vi "demo.vi"() -> ()   [LabVIEW 2017]
uses:
  globe.vi
  Instance           7 12Saved   demo .vi
  Instance           3 12Saved   demo .vi
  Instance           6 12Saved   demo .vi
  Instance           4 12Saved   demo .vi
  Instance           5 12Saved   demo .vi
  Instance           2 12Saved   demo .vi
  Instance           1 12Saved   demo .vi
  bin/ControlCAN.dll
panel:
  in  "清除定时发送":bool
  in  "定时发送":bool
  out "DBC界面":bool
  in  "DBC发送界面":bool
  in  "设备类型":u32(ring)=1 items=["PCI5121"=1, "PCI9810"=2, "USBCAN1"=3, "USBCAN2"=4, "PCI9820"=5, "PCI5110"=7, "PC104CAN"=11, "CANETUDP"=12, "PCI9840B"=14, "PC104C2"=15, "PCI9820I"=16, "CANETTCP"=17, "PCIE9221"=24, "PCI5010U"=19, "USBCAN_E_U"=20, "USBCAN_2E_U"=21, "CANalyst-II+"=10021, "PCI5020U"=22, "PCIE9120I"=27, "PCIE9110I"=28, "PCIE9140I"=29]
  in  "总线利用率":bool
  in  "索引":u32(ring) items=["0", "1", "2", "3", "4", "5", "6", "7", "8"]
  in  "Radio_Baud(E_U)":bool=TRUE
  in  "寄存器":u32 format="0x%08x"
  in  "Radio_Baud":bool=TRUE
  in  "Baud":u32(ring) caption="波特率" items=["5Kbps", "10Kbps", "20Kbps", "40Kbps", "50Kbps", "80Kbps", "100Kbps", "125Kbps", "200Kbps", "250Kbps", "400Kbps", "500Kbps", "666Kbps", "800Kbps", "1000Kbps"]
  out "VCI_CAN_OBJ_TN":T1(array[cluster])
  out "VCI_CAN_OBJ_RN":T1(array[cluster])
  in  "arraylen":u32
  in  "一次发送帧数":u32
  out "type":u8[](array[numeric])
  in  "本机端口":u32
  in  "本机类型":enum32{"Radio Selection 1", "Radio Selection 2"}(radio)
  in  "CANET 端口":u32
  in  "CANET IP":string
  out "VCI_FILTER_RECORD":cluster{"ExtFrame":u32, "Start":u32, "End":u32}
  in  "e-u-baud":cluster{"数值":u32}
  in  "滤波模式":u32(ring) items=["标准帧滤波", "扩展帧滤波", "禁能滤波"]
  in  "滤波起始ID":u32
  in  "滤波结束ID":u32
  in  "Baud(E_U)":u32(ring) caption="波特率" items=["1000Kbps"=393219, "800Kbps"=393220, "500Kbps"=393223, "250Kbps"=1835016, "125Kbps"=1835025, "100Kbps"=1441827, "50Kbps"=1835052, "20Kbps"=1441971, "10Kbps"=1835232, "5Kbps"=1835457]
  in  "SEND_NCAN":bool
  out "VCI_CAN_OBJ_T_N":T1(array[cluster])
  out "接收缓冲区":u32
  in  "GetStatus":bool
  in  "GetErrorInfo":bool
  in  "GetBoardInfo":bool
  in  "Clear Buffer":bool
  in  "Transmit":bool
  out "VCI_BOARD_INFO":T2
  out "VCI_ERR_INFO":T3
  out "VCI_CAN_STATUS":T4
  in  "模式":u8(ring) items=["正常", "只听"]
  in  "滤波方式":u8(ring) items=["双滤波", "单滤波"]
  in  "BTR1":u8=20 format="0x%02x"
  in  "BTR0":u8 format="0x%02x"
  in  "屏蔽码":u32=4294967295 format="0x%08x"
  in  "验收码":u32 format="0x%08x"
  in  "ID":u32 format="0x%08x"
  in  "数据输入":string
  in  "TREvent":T5={"Tx_Or_Rx"=FALSE, "VCI_CAN_OBJ"={"ID"=0, "TimeStamp"=0, "TimeFlag"=0, "SendType"=1, "RemoteFlag"=0, "ExternFlag"=0, "DataLen"=8, 0, 0, 0, 0, 0, 0, 0, 0, 0, 0, 0}, "VCI_CAN_OBJ_N"=[], "Num"=0}
  out "stop 2":bool
  out "Num Rows":u32
  out "TRCount":u32
  out "VCI_CAN_OBJ_R":T6={"ID"=0, "TimeStamp"=0, "TimeFlag"=0, "SendType"=1, "RemoteFlag"=0, "ExternFlag"=0, "DataLen"=8, 0, 0, 0, 0, 0, 0, 0, 0, 0, 0, 0}
  out "VCI_CAN_OBJ_T":T6={"ID"=0, "TimeStamp"=0, "TimeFlag"=0, "SendType"=1, "RemoteFlag"=0, "ExternFlag"=0, "DataLen"=8, 0, 0, 0, 0, 0, 0, 0, 0, 0, 0, 0}
  out "VCI_INIT_CONFIG":T7={"AccCode"=0, "AccMask"=4294967295, "Reserved"=0, "Filter"=1, "Timing0"=0, "Timing1"=20, "Mode"=0}
  out "CANStartup":bool
  in  "DeviceOpen":bool
  in  "OpenDevice":bool
  in  "帧格式":u8(ring) items=["数据帧", "远程帧"]
  in  "帧类型":u8(ring) items=["标准帧", "扩展帧"]
  in  "发送类型":u8(ring) items=["正常发送", "单次发送", "自发自收", "单次自发自收"]
  in  "设备类型值":u32(ring)=1 items=["PCI5121"=1, "PCI9810"=2, "USBCAN1"=3, "USBCAN2"=4, "PCI9820"=5, "PCI5110"=7, "PC104CAN"=11, "CANETUDP"=12, "PCI9840B"=14, "PC104C2"=15, "PCI9820I"=16, "CANETTCP"=17, "PCIE9221"=24, "PCI5010U"=19, "USBCAN_E_U"=20, "USBCAN_2E_U"=21, "PCI5020U"=22, "PCIE9120I"=27, "PCIE9110I"=28, "PCIE9140I"=29]
  in  "ResetCAN":bool
  in  "StartCAN":bool
  in  "CAN 通道":u32(ring) items=["0", "1"]
  in  "stop":bool
  out "Multicolumn Listbox":i32(listbox)
  # "CANET 设备特殊设置"
  # "_U系列特殊设置"
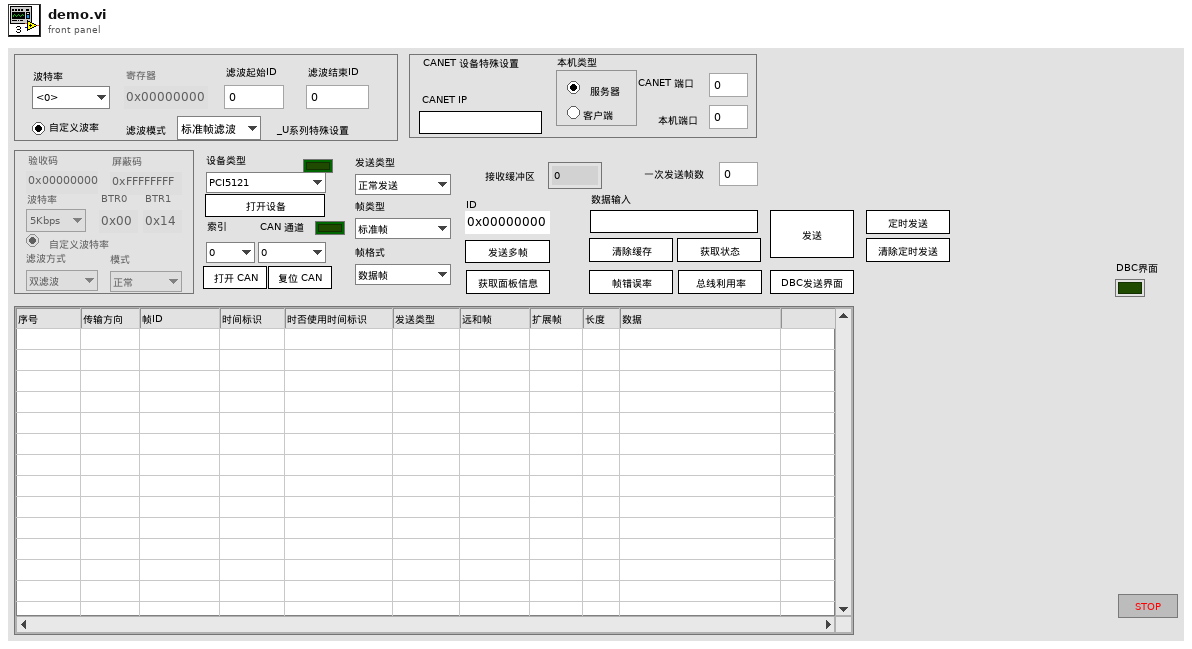
[diagram p1: front panel]
types:
  T1 = cluster{"ID":u32, "TimeStamp":u32, "TimeFlag":u8, "SendType":u8, "RemoteFlag":u8, "ExternFlag":u8, "DataLen":u8, u8, u8, u8, u8, u8, u8, u8, u8, u8, u8, u8}[]
  T2 = cluster{"hw_Version":u16, "fw_Version":u16, "dr_Version":u16, "in_Version":u16, "irq_Num":u16, "can_Num":u8, "str_Serial_Num 0":i8, "str_Serial_Num 1":i8, "str_Serial_Num 2":i8, "str_Serial_Num 3":i8, "str_Serial_Num 4":i8, "str_Serial_Num 5":i8, "str_Serial_Num 6":i8, "str_Serial_Num 7":i8, "str_Serial_Num 8":i8, "str_Serial_Num 9":i8, "str_Serial_Num 10":i8, "str_Serial_Num 11":i8, "str_Serial_Num 12":i8, "str_Serial_Num 13":i8, "str_Serial_Num 14":i8, "str_Serial_Num 15":i8, "str_Serial_Num 16":i8, "str_Serial_Num 17":i8, "str_Serial_Num 18":i8, "str_Serial_Num 19":i8, "str_hw_Type 0":i8, "str_hw_Type 1":i8, "str_hw_Type 2":i8, "str_hw_Type 3":i8, "str_hw_Type 4":i8, "str_hw_Type 5":i8, "str_hw_Type 6":i8, "str_hw_Type 7":i8, "str_hw_Type 8":i8, "str_hw_Type 9":i8, "str_hw_Type 10":i8, "str_hw_Type 11":i8, "str_hw_Type 12":i8, "str_hw_Type 13":i8, "str_hw_Type 14":i8, "str_hw_Type 15":i8, "str_hw_Type 16":i8, "str_hw_Type 17":i8, "str_hw_Type 18":i8, "str_hw_Type 19":i8, "str_hw_Type 20":i8, "str_hw_Type 21":i8, "str_hw_Type 22":i8, "str_hw_Type 23":i8, "str_hw_Type 24":i8, "str_hw_Type 25":i8, "str_hw_Type 26":i8, "str_hw_Type 27":i8, "str_hw_Type 28":i8, "str_hw_Type 29":i8, "str_hw_Type 30":i8, "str_hw_Type 31":i8, "str_hw_Type 32":i8, "str_hw_Type 33":i8, "str_hw_Type 34":i8, "str_hw_Type 35":i8, "str_hw_Type 36":i8, "str_hw_Type 37":i8, "str_hw_Type 38":i8, "str_hw_Type 39":i8, "Reserved 0":u16, "Reserved 1":u16, "Reserved 2":u16, "Reserved 3":u16}
  T3 = cluster{"ErrCode":u32, "Passive_ErrData0":u8, "Passive_ErrData1":u8, "Passive_ErrData2":u8, "ArLost_ErrData":u8}
  T4 = cluster{"ErrInterrupt":u8, "regMode":u8, "regStatus":u8, "regALCapture":u8, "regECCapture":u8, "regEWLimit":u8, "regRECounter":u8, "regTECounter":u8, "Reserved":u32}
  T5 = cluster{"Tx_Or_Rx":bool, "VCI_CAN_OBJ":cluster{"ID":u32, "TimeStamp":u32, "TimeFlag":u8, "SendType":u8, "RemoteFlag":u8, "ExternFlag":u8, "DataLen":u8, u8, u8, u8, u8, u8, u8, u8, u8, u8, u8, u8}, "VCI_CAN_OBJ_N":cluster{"ID":u32, "TimeStamp":u32, "TimeFlag":u8, "SendType":u8, "RemoteFlag":u8, "ExternFlag":u8, "DataLen":u8, u8, u8, u8, u8, u8, u8, u8, u8, u8, u8, u8}[], "Num":u32}
  T6 = cluster{"ID":u32, "TimeStamp":u32, "TimeFlag":u8, "SendType":u8, "RemoteFlag":u8, "ExternFlag":u8, "DataLen":u8, u8, u8, u8, u8, u8, u8, u8, u8, u8, u8, u8}
  T7 = cluster{"AccCode":u32, "AccMask":u32, "Reserved":u32, "Filter":u8, "Timing0":u8, "Timing1":u8, "Mode":u8}
  T8 = cluster{bool, "VCI_CAN_OBJ_R":cluster{"ID":u32, "TimeStamp":u32, "TimeFlag":u8, "SendType":u8, "RemoteFlag":u8, "ExternFlag":u8, "DataLen":u8, u8, u8, u8, u8, u8, u8, u8, u8, u8, u8, u8}, "pReceive":cluster{"ID":u32, "TimeStamp":u32, "TimeFlag":u8, "SendType":u8, "RemoteFlag":u8, "ExternFlag":u8, "DataLen":u8, u8, u8, u8, u8, u8, u8, u8, u8, u8, u8, u8}[], "return type":u32}
  T9 = enum8{"Enabled", "Disabled", "Disabled and Grayed Out"}
  T10 = cluster{"[0]":u32, "[1]":u32, "[2]":u32, "[3]":u32, "[4]":u32, "[5]":u32, "[6]":u32, "[7]":u32, "[8]":u32}
  T11 = cluster{"验收码":u32, "屏蔽码":u32, u32, "滤波方式":u8, "BTR0":u8, "BTR1":u8, "模式":u8}
  T12 = cluster{"ID":u32, u32, u8, "发送类型":u8, "帧格式":u8, "帧类型":u8, i32, "[0]":u32, "[1]":u32, "[2]":u32, "[3]":u32, "[4]":u32, "[5]":u32, "[6]":u32, "[7]":u32, u8, u8, u8}
  T13 = cluster{u8, u8, u8, u8, u32, "VCI_CAN_OBJ_T":cluster{"ID":u32, "TimeStamp":u32, "TimeFlag":u8, "SendType":u8, "RemoteFlag":u8, "ExternFlag":u8, "DataLen":u8, u8, u8, u8, u8, u8, u8, u8, u8, u8, u8, u8}}
  T14 = cluster{bool, "VCI_CAN_OBJ_T":cluster{"ID":u32, "TimeStamp":u32, "TimeFlag":u8, "SendType":u8, "RemoteFlag":u8, "ExternFlag":u8, "DataLen":u8, u8, u8, u8, u8, u8, u8, u8, u8, u8, u8, u8}, cluster{"ID":u32, "TimeStamp":u32, "TimeFlag":u8, "SendType":u8, "RemoteFlag":u8, "ExternFlag":u8, "DataLen":u8, u8, u8, u8, u8, u8, u8, u8, u8, u8, u8, u8}[], "return type":u32}
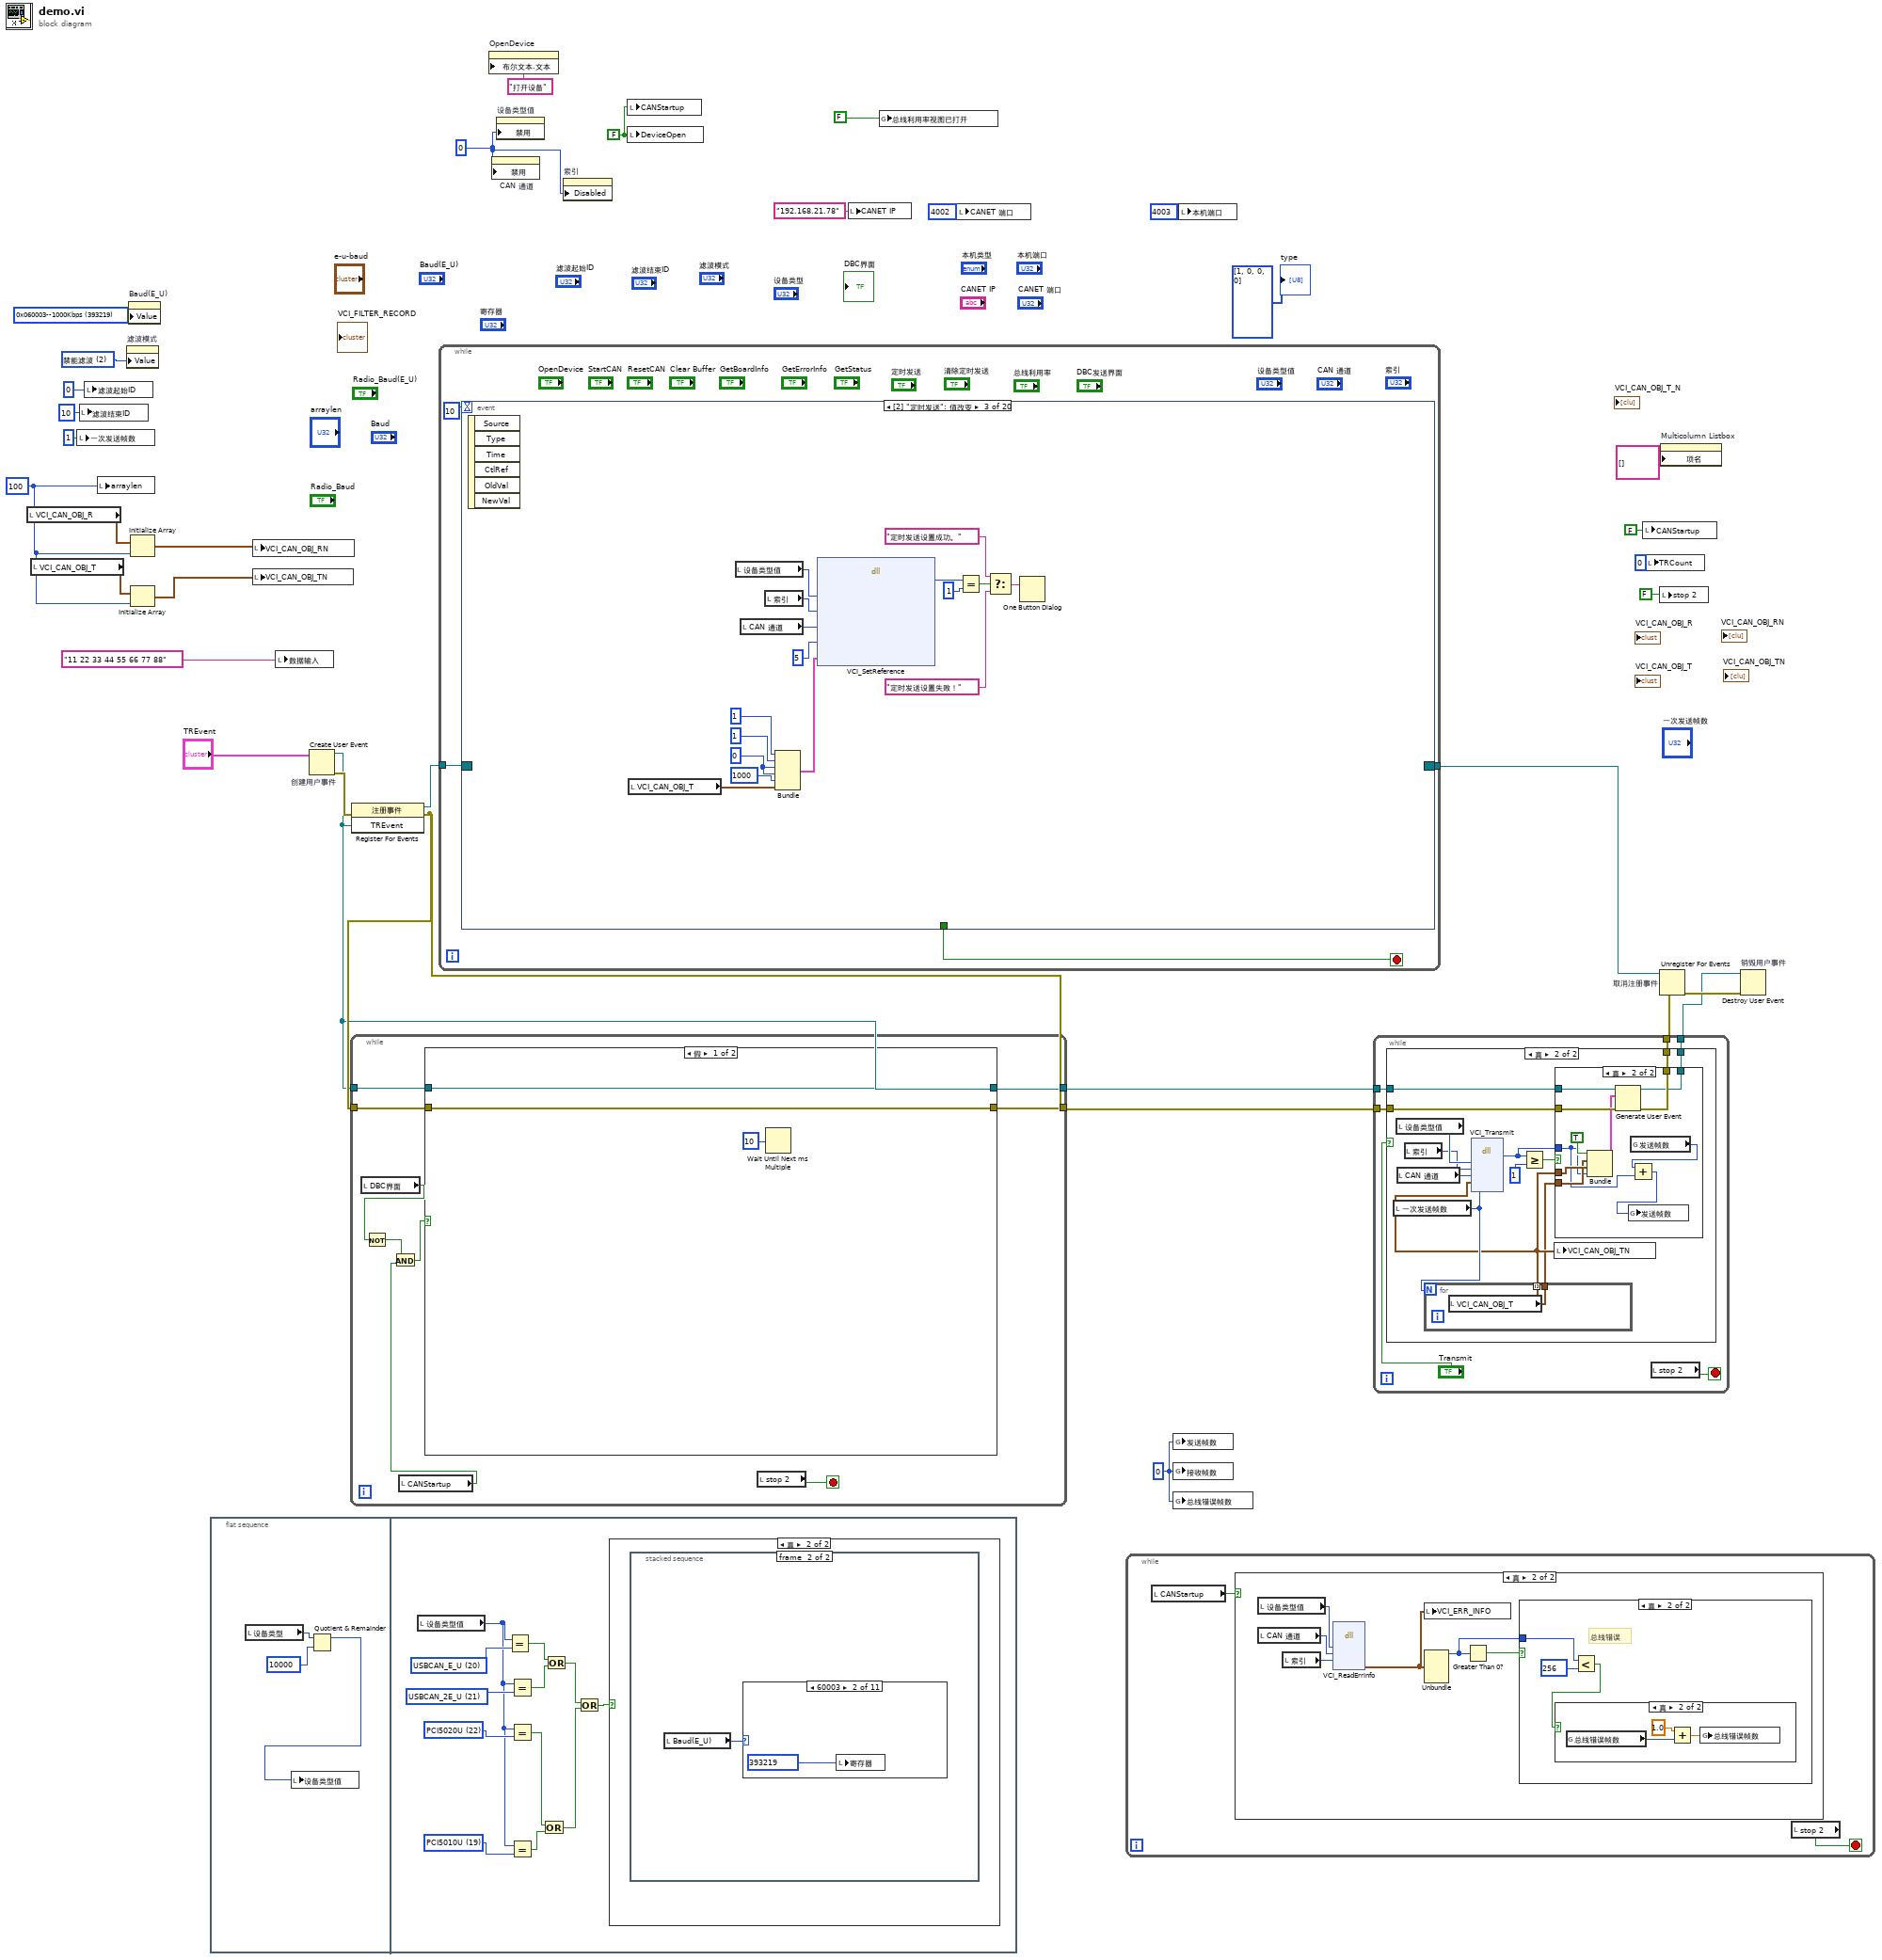
[diagram p0: block diagram]
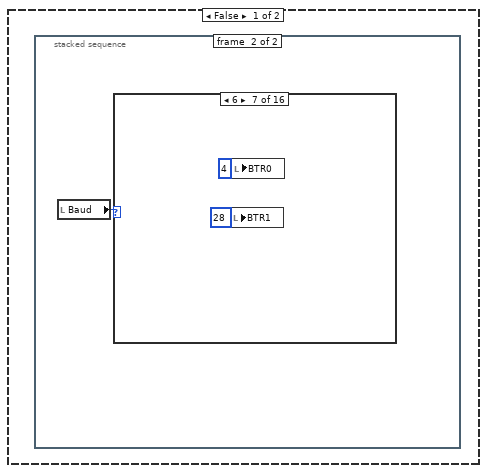
[diagram p2: hidden frame]
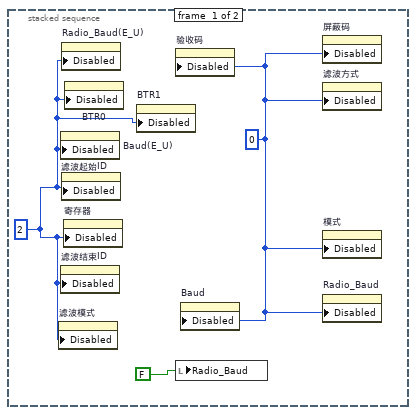
[diagram p3: hidden frame]
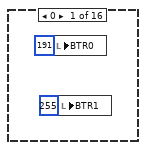
[diagram p4: hidden frame]
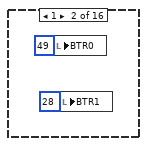
[diagram p5: hidden frame]
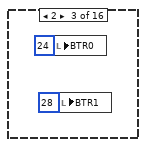
[diagram p6: hidden frame]
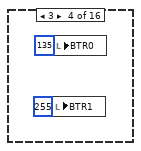
[diagram p7: hidden frame]
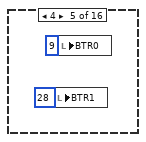
[diagram p8: hidden frame]
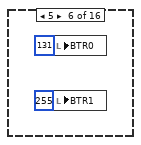
[diagram p9: hidden frame]
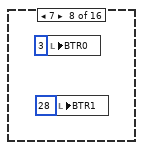
[diagram p10: hidden frame]
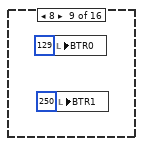
[diagram p11: hidden frame]
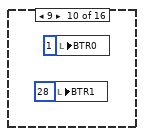
[diagram p12: hidden frame]
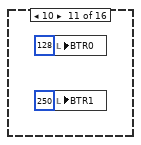
[diagram p13: hidden frame]
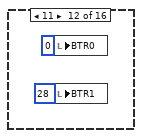
[diagram p14: hidden frame]
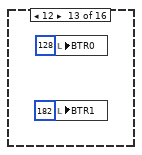
[diagram p15: hidden frame]
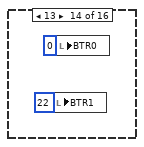
[diagram p16: hidden frame]
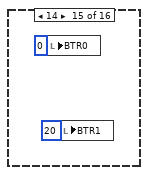
[diagram p17: hidden frame]
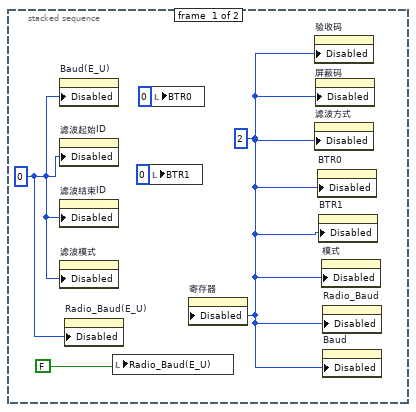
[diagram p19: hidden frame]
diagram:
  w2 = u8 0 ("Disabled")
  w4 = FALSE ("DeviceOpen")
  w5 = 0
  w12 = u32 100 ("arraylen")
  w20 = u32 2 items=["标准帧滤波", "扩展帧滤波", "禁能滤波"] ("fiter_mode")
  w21 = u32 393219 items=["0x060003--1000Kbps"=393219, "0x060004--800Kbps"=393220, "0x060007--500Kbps"=393223, "0x1C0008--250Kbps"=1835016, "0x1C0011--125Kbps"=1835025, "0x160023--100Kbps"=1441827, "0x1C002C--50Kbps"=1835052, "0x1600B3--20Kbps"=1441971, "0x1C00E0--10Kbps"=1835232, "0x1C01C1--5Kbps"=1835457] ("E-U_baud")
  n1 = local read "VCI_CAN_OBJ_R"() -> (w15:T6)
  n2 = local read "VCI_CAN_OBJ_T"() -> (w13:T6)
  n3 = local write "一次发送帧数"(u32 1 ("一次发送帧数")) -> ()
  n4 = local write "滤波结束ID"(u32 10 ("fiter_endid")) -> ()
  n5 = local write "滤波起始ID"(u32 0 ("fiter_startid")) -> ()
  n6 = local write "arraylen"(w12) -> ()
  n7 = property on="滤波模式" class="Ring (严格)"("Value"=w20) -> ()  [unwired: 2 in, 2 out]
  n8 = property on="Baud(E_U)" class="Ring (严格)"("Value"=w21) -> ()  [unwired: 2 in, 2 out]
  n9 = Initialize Array(w15, w12) -> (w14:T1)
  n10 = Initialize Array(w13, w12) -> (w11:T1)
  n11 = flat-sequence {
    frame #0 {
      n12 = local read "设备类型"() -> (w36:u32)
      n13 = Quotient & Remainder(x=w36, y=10000) -> (x-y*floor(x/y)=w34:u32)  [unwired: 1 out]
      n14 = local write "设备类型值"(w34) -> ()
    }
    frame #1 {
      w45 = u32 19 items=["PCI5121"=1, "PCI9810"=2, "USBCAN1"=3, "USBCAN2"=4, "PCI9820"=5, "PCI5110"=7, "CANLite(mini)"=8, "ISA9620"=9, "ISA5420"=10, "PC104CAN"=11, "DNP9810"=13, "PCI9840B"=14, "PC104C2"=15, "PCI9820I"=16, "pec9920"=18, "PCI5010U"=19, "USBCAN_E_U"=20, "USBCAN_2E_U"=21, "PCI5020U"=22, ""=0] ("DeviceType")
      w46 = u32 22 items=["PCI5121"=1, "PCI9810"=2, "USBCAN1"=3, "USBCAN2"=4, "PCI9820"=5, "PCI5110"=7, "CANLite(mini)"=8, "ISA9620"=9, "ISA5420"=10, "PC104CAN"=11, "DNP9810"=13, "PCI9840B"=14, "PC104C2"=15, "PCI9820I"=16, "pec9920"=18, "PCI5010U"=19, "USBCAN_E_U"=20, "USBCAN_2E_U"=21, "PCI5020U"=22, ""=0] ("DeviceType")
      w47 = u32 21 items=["PCI5121"=1, "PCI9810"=2, "USBCAN1"=3, "USBCAN2"=4, "PCI9820"=5, "PCI5110"=7, "CANLite(mini)"=8, "ISA9620"=9, "ISA5420"=10, "PC104CAN"=11, "DNP9810"=13, "PCI9840B"=14, "PC104C2"=15, "PCI9820I"=16, "pec9920"=18, "USBCAN_E_U"=20, "USBCAN_2E_U"=21, ""=0] ("DeviceType")
      w48 = u32 20 items=["PCI5121"=1, "PCI9810"=2, "USBCAN1"=3, "USBCAN2"=4, "PCI9820"=5, "PCI5110"=7, "CANLite(mini)"=8, "ISA9620"=9, "ISA5420"=10, "PC104CAN"=11, "DNP9810"=13, "PCI9840B"=14, "PC104C2"=15, "PCI9820I"=16, "pec9920"=18, "USBCAN_E_U"=20, "USBCAN_2E_U"=21, ""=0] ("DeviceType")
      n15 = local read "设备类型值"() -> (w44:u32)
      n16 = Equal?(x=w44, y=w48) -> (x = y?=w43:bool)
      n17 = Equal?(x=w44, y=w47) -> (x = y?=w42:bool)
      n18 = Equal?(x=w44, y=w46) -> (x = y?=w41:bool)
      n19 = Equal?(x=w44, y=w45) -> (x = y?=w40:bool)
      n20 = Or(x=w41, y=w40) -> (x .or. y?=w38:bool)
      n21 = Or(x=w43, y=w42) -> (x .or. y?=w39:bool)
      n22 = Or(x=w39, y=w38) -> (x .or. y?=w37:bool)
      n23 = case shown="真" w37 {
        frame False {
          n24 = stacked-sequence {
            frame #0 {
              w51 = 0
              w50 = 2
              n25 = property on="滤波模式" class="Ring (严格)"("Disabled"=w50) -> ()  [unwired: 2 in, 2 out]
              n26 = property on="Baud(E_U)" class="Ring (严格)"("Disabled"=w50) -> ()  [unwired: 2 in, 2 out]
              n27 = property on="滤波结束ID" class="DigNum (严格)"("Disabled"=w50) -> ()  [unwired: 2 in, 2 out]
              n28 = property on="Radio_Baud(E_U)" class="Bool (严格)"("Disabled"=w50) -> ()  [unwired: 2 in, 2 out]
              n29 = property on="滤波起始ID" class="DigNum (严格)"("Disabled"=w50) -> ()  [unwired: 2 in, 2 out]
              n30 = property on="寄存器" class="DigNum (严格)"("Disabled"=w50) -> ()  [unwired: 2 in, 2 out]
              n31 = property on="BTR0" class="DigNum (严格)"("Disabled"=w50) -> ()  [unwired: 2 in, 2 out]
              n32 = property on="BTR1" class="DigNum (严格)"("Disabled"=w50) -> ()  [unwired: 2 in, 2 out]
              n33 = property on="验收码" class="DigNum (严格)"("Disabled"=w51) -> ()  [unwired: 2 in, 2 out]
              n34 = local write "Radio_Baud"(FALSE) -> ()
              n35 = property on="Baud" class="Ring (严格)"("Disabled"=w51) -> ()  [unwired: 2 in, 2 out]
              n36 = property on="屏蔽码" class="DigNum (严格)"("Disabled"=w51) -> ()  [unwired: 2 in, 2 out]
              n37 = property on="滤波方式" class="Ring (严格)"("Disabled"=w51) -> ()  [unwired: 2 in, 2 out]
              n38 = property on="模式" class="Ring (严格)"("Disabled"=w51) -> ()  [unwired: 2 in, 2 out]
              n39 = property on="Radio_Baud" class="Bool (严格)"("Disabled"=w51) -> ()  [unwired: 2 in, 2 out]
            }
            frame #1 {
              n40 = local read "Baud"() -> (w52:u32)
              n41 = case shown="6" w52 {
                frame 0 {
                  n42 = local write "BTR0"(u8 191 ("BTR0")) -> ()
                  n43 = local write "BTR1"(u8 255 ("BTR1")) -> ()
                }
                frame 1 {
                  n44 = local write "BTR0"(u8 49 ("BTR0")) -> ()
                  n45 = local write "BTR1"(u8 28 ("BTR1")) -> ()
                }
                frame 2 {
                  n46 = local write "BTR0"(u8 24 ("BTR0")) -> ()
                  n47 = local write "BTR1"(u8 28 ("BTR1")) -> ()
                }
                frame 3 {
                  n48 = local write "BTR1"(u8 255 ("BTR1")) -> ()
                  n49 = local write "BTR0"(u8 135 ("BTR0")) -> ()
                }
                frame 4 {
                  n50 = local write "BTR1"(u8 28 ("BTR1")) -> ()
                  n51 = local write "BTR0"(u8 9 ("BTR0")) -> ()
                }
                frame 5 {
                  n52 = local write "BTR0"(u8 131 ("BTR0")) -> ()
                  n53 = local write "BTR1"(u8 255 ("BTR1")) -> ()
                }
                frame 6 {
                  n54 = local write "BTR1"(u8 28 ("BTR1")) -> ()
                  n55 = local write "BTR0"(u8 4 ("BTR0")) -> ()
                }
                frame 7 {
                  n56 = local write "BTR0"(u8 3 ("BTR0")) -> ()
                  n57 = local write "BTR1"(u8 28 ("BTR1")) -> ()
                }
                frame 8 {
                  n58 = local write "BTR0"(u8 129 ("BTR0")) -> ()
                  n59 = local write "BTR1"(u8 250 ("BTR1")) -> ()
                }
                frame 9 {
                  n60 = local write "BTR1"(u8 28 ("BTR1")) -> ()
                  n61 = local write "BTR0"(u8 1 ("BTR0")) -> ()
                }
                frame 10 {
                  n62 = local write "BTR0"(u8 128 ("BTR0")) -> ()
                  n63 = local write "BTR1"(u8 250 ("BTR1")) -> ()
                }
                frame 11 {
                  n64 = local write "BTR0"(u8 0 ("BTR0")) -> ()
                  n65 = local write "BTR1"(u8 28 ("BTR1")) -> ()
                }
                frame 12 {
                  n66 = local write "BTR0"(u8 128 ("BTR0")) -> ()
                  n67 = local write "BTR1"(u8 182 ("BTR1")) -> ()
                }
                frame 13 {
                  n68 = local write "BTR1"(u8 22 ("BTR1")) -> ()
                  n69 = local write "BTR0"(u8 0 ("BTR0")) -> ()
                }
                frame 14 {
                  n70 = local write "BTR0"(u8 0 ("BTR0")) -> ()
                  n71 = local write "BTR1"(u8 20 ("BTR1")) -> ()
                }
                frame 15, Default {
                }
              }
            }
          }
        }
        frame True {
          n72 = stacked-sequence {
            frame #0 {
              w85 = 0
              w83 = 2
              n73 = property on="Baud(E_U)" class="Ring (严格)"("Disabled"=w85) -> ()  [unwired: 2 in, 2 out]
              n74 = property on="滤波起始ID" class="DigNum (严格)"("Disabled"=w85) -> ()  [unwired: 2 in, 2 out]
              n75 = property on="滤波结束ID" class="DigNum (严格)"("Disabled"=w85) -> ()  [unwired: 2 in, 2 out]
              n76 = property on="滤波模式" class="Ring (严格)"("Disabled"=w85) -> ()  [unwired: 2 in, 2 out]
              n77 = property on="Radio_Baud(E_U)" class="Bool (严格)"("Disabled"=w85) -> ()  [unwired: 2 in, 2 out]
              n78 = local write "Radio_Baud(E_U)"(FALSE) -> ()
              n79 = local write "BTR1"(u8 0 ("BTR1")) -> ()
              n80 = local write "BTR0"(u8 0 ("BTR0")) -> ()
              n81 = property on="寄存器" class="DigNum (严格)"("Disabled"=w83) -> ()  [unwired: 2 in, 2 out]
              n82 = property on="验收码" class="DigNum (严格)"("Disabled"=w83) -> ()  [unwired: 2 in, 2 out]
              n83 = property on="滤波方式" class="Ring (严格)"("Disabled"=w83) -> ()  [unwired: 2 in, 2 out]
              n84 = property on="屏蔽码" class="DigNum (严格)"("Disabled"=w83) -> ()  [unwired: 2 in, 2 out]
              n85 = property on="BTR0" class="DigNum (严格)"("Disabled"=w83) -> ()  [unwired: 2 in, 2 out]
              n86 = property on="BTR1" class="DigNum (严格)"("Disabled"=w83) -> ()  [unwired: 2 in, 2 out]
              n87 = property on="模式" class="Ring (严格)"("Disabled"=w83) -> ()  [unwired: 2 in, 2 out]
              n88 = property on="Radio_Baud" class="Bool (严格)"("Disabled"=w83) -> ()  [unwired: 2 in, 2 out]
              n89 = property on="Baud" class="Ring (严格)"("Disabled"=w83) -> ()  [unwired: 2 in, 2 out]
            }
            frame #1 {
              n90 = local read "Baud(E_U)"() -> (w88:u32)
              n91 = case shown="60003" w88 {
                frame 286331153, Default {
                }
                frame 393219 {
                  n92 = local write "寄存器"(393219) -> ()
                }
                frame 393220 {
                  n93 = local write "寄存器"(393220) -> ()
                }
                frame 393223 {
                  n94 = local write "寄存器"(393223) -> ()
                }
                frame 1835016 {
                  n95 = local write "寄存器"(1835016) -> ()
                }
                frame 1835025 {
                  n96 = local write "寄存器"(1835025) -> ()
                }
                frame 1441827 {
                  n97 = local write "寄存器"(1441827) -> ()
                }
                frame 1835052 {
                  n98 = local write "寄存器"(1835052) -> ()
                }
                frame 1441971 {
                  n99 = local write "寄存器"(1441971) -> ()
                }
                frame 1835232 {
                  n100 = local write "寄存器"(1835232) -> ()
                }
                frame 1835457 {
                  n101 = local write "寄存器"(1835457) -> ()
                }
              }
            }
          }
        }
      }
    }
  }
  n102 = local write "VCI_CAN_OBJ_RN"(w14) -> ()
  n103 = local write "VCI_CAN_OBJ_TN"(w11) -> ()
  n104 = local write "数据输入"("11 22 33 44 55 66 77 88" ("Data Input")) -> ()
  n105 = Create User Event "创建用户事件"(user event datatype="TREvent") -> (user event=w6:refnum<user-event>, error out=w30:errorcluster)  [unwired: 1 in]
  n106 = register-events(error in=w30, w6) -> (reference out=w27:refnum<event-registration>, error out=w23:errorcluster)  [unwired: 1 in]
  n107 = while {
    tunnel: w6 -> [w107]
    tunnel: w23 -> [w106]
    tunnel: [w105] -> _
    tunnel: [w104] -> _
    stop <- w103 stop-if-true
    n108 = local read "DBC界面"() -> (w102:bool)
    n109 = Not(x=w102) -> (.not. x?=w101:bool)
    n110 = local read "CANStartup"() -> (w100:bool)
    n111 = And(x=w101, y=w100) -> (x .and. y?=w99:bool)
    n112 = case shown="假" w99 {
      tunnel: w107 -> [w110 w124]
      tunnel: w106 -> [w109 w123]
      tunnel: [w110 w122] -> w105
      tunnel: [w109 w121] -> w104
      frame False {
        n113 = Wait Until Next ms Multiple(millisecond multiple=u32 10) -> ()  [unwired: 1 out]
      }
      frame True {
        n114 = local read "CAN 通道"() -> (w117:u32)
        n115 = local read "设备类型值"() -> (w119:u32)
        n116 = local read "索引"() -> (w118:u32)
        n117 = dll-call lib="E:/Project/CANMaster/LabView/ControlCAN_labview/bin/ControlCAN.dll" fn="VCI_GetReceiveNum"("DeviceType"=w119, "DeviceInd"=w118, "CANInd"=w117) -> ("return type"=w111:u32)  [unwired: 6 in, 2 out]
        n118 = Greater Or Equal?(x=w111, y=u32 1) -> (x >= y?=w112:bool)
        n119 = case shown="真" w112 {
          tunnel: [_ w128] -> w116
          tunnel: [_ w127] -> w115
          tunnel: [_ w126] -> w114
          tunnel: w111 -> [_ w125]
          frame False {
          }
          frame True {
            n120 = local read "VCI_CAN_OBJ_RN"() -> (w132:T1)
            n121 = local read "设备类型值"() -> (w131:u32)
            n122 = local read "CAN 通道"() -> (w130:u32)
            n123 = local read "索引"() -> (w134:u32)
            n124 = dll-call lib="E:/Project/CANMaster/LabView/ControlCAN_labview/bin/ControlCAN.dll" fn="VCI_Receive"("DeviceType"=w131, "DeviceInd"=w134, "CANInd"=w130, "pReceive"=w132, "Len"=w125, "WaitTime"=100) -> ("return type"=w128:u32, "pReceive"=w126:T1)  [unwired: 8 in, 2 out]
            n125 = local write "VCI_CAN_OBJ_RN"(w126) -> ()
            n126 = Greater Or Equal?(x=w128, y=u32 1) -> (x >= y?=w127:bool)
          }
        }
        n127 = local read "VCI_CAN_OBJ_R"() -> (w120:T6)
        n128 = case shown="真" w115 {
          tunnel: w124 -> [w136 w147]
          tunnel: w123 -> [w135 w146]
          tunnel: [w136 w145] -> w122
          tunnel: [w135 w144] -> w121
          tunnel: w114 -> [_ w141]
          tunnel: w116 -> [_ w138]
          tunnel: w120 -> [_ w140]
          frame False {
          }
          frame True {
            n129 = Bundle(FALSE, "VCI_CAN_OBJ_R"=w140, "pReceive"=w141, "return type"=w138) -> (w142:T8)  [unwired: 1 out]
            n130 = Generate User Event "产生用户事件"(user event=w147, event data cluster=w142, error in=w146) -> (user event out=w145:refnum<user-event>, error out=w144:errorcluster)  [unwired: 1 in]
            n131 = global read "globe.vi" "接收帧数"() -> (w139:u32)
            n132 = Add(x=w139, y=w138) -> (x+y=w137:u32)
            n133 = global write "globe.vi" "接收帧数"(w137) -> ()
          }
        }
      }
    }
    n134 = local read "stop 2"() -> (w103:bool)
  }
  n135 = while {
    tunnel: w27 -> [w151]
    tunnel: [w150] -> w26
    stop <- w148 stop-if-true
    n136 = event shown="[2] \"定时发送\": 值改变" {
      selector: w151 -> [_ _ _ _ _ _ _ _ _ _ _ _ _ _ _ _ _ _ _ _]
      dyn-events: [_ _ _ _ _ _ _ _ _ _ _ _ _ _ _ _ _ _ _ _] -> w150
      timeout: 10 -> [_ _ _ _ _ _ _ _ _ _ _ _ _ _ _ _ _ _ _ _]
      tunnel: [_ _ _ _ _ _ w286 _ _ _ _ _ _ _ _ _ _ _ _ _] -> w148
      event Timeout {
        w188 = u8 0
        w176 = u32 0
        n137 = event-data() -> ()  [unwired: 2 out]
        n138 = local read "索引"() -> (w152:u32)
        n139 = local read "滤波结束ID"() -> (w154:u32)
        n140 = local read "设备类型值"() -> (w162:u32)
        n141 = local read "滤波起始ID"() -> (w155:u32)
        n142 = local read "CAN 通道"() -> (w159:u32)
        n143 = local read "滤波模式"() -> (w157:u32)
        n144 = for {
          N: 8 -> [_]
          tunnel: "数据输入" -> [w203]
          tunnel: [w206] -> w174 mode=indexing
          tunnel: [w191] -> w172
          i -> [w196]
          n145 = Multiply(x=3, y=w196) -> (x*y=w209:i32)
          n146 = String Length(string=w203) -> (length=w202:i32)
          n147 = String Subset(string=w203, offset (0)=w209, length (rest)=2 ("length (rest)")) -> (substring=w200:string)
          n148 = Quotient & Remainder(x=w202, y=3) -> (x-y*floor(x/y)=w198:i32, floor(x/y)=w194:i32)
          n149 = Equal To 0?(x=w198) -> (x = 0?=w197:bool)
          n150 = Increment(x=w194) -> (x+1=w195:i32)
          n151 = Hex Digit?(1:w200) -> (0:w204:bool)
          n152 = Select(t=w194, s=w197, f=w195) -> (s? t:f=w193:i32)
          n153 = Select(t=w200, s=w204, f="00" ("t")) -> (s? t:f=w205:string)
          n154 = Quotient & Remainder(x=w193, y=9) -> (x-y*floor(x/y)=w191:i32)  [unwired: 1 out]
          n155 = Scan From String(format string="%2x ", input string=w205) -> (output 1=w206:u32)  [unwired: 2 in, 4 out]
        }
        n156 = dll-call lib="E:/Project/CANMaster/LabView/ControlCAN_labview/bin/ControlCAN.dll" fn="VCI_GetReceiveNum"("DeviceType"=w162, "DeviceInd"=w152, "CANInd"=w159) -> (→"接收缓冲区":u32)  [unwired: 6 in, 2 out]
        n157 = Bundle("滤波模式"=w157, "滤波起始ID"=w155, "滤波结束ID"=w154) -> (w156:cluster{"滤波模式":u32, "滤波起始ID":u32, "滤波结束ID":u32})  [unwired: 1 out]
        n158 = local write "VCI_FILTER_RECORD"(w156) -> ()
        n159 = Array To Cluster(array=w174) -> (cluster=w173:T10)
        n160 = To Unsigned Byte Integer(number=w176) -> (unsigned 8bit integer=w175:u8)
        n161 = Unbundle(w173) -> ("[0]"=w180:u32, "[1]"=w181:u32, "[2]"=w182:u32, "[3]"=w183:u32, "[4]"=w184:u32, "[5]"=w185:u32, "[6]"=w186:u32, "[7]"=w187:u32)  [unwired: 1 out]
        n162 = Bundle("验收码"="验收码", "屏蔽码"="屏蔽码", u32 0, "滤波方式"="滤波方式", "BTR0"="BTR0", "BTR1"="BTR1", "模式"="模式") -> (→"VCI_INIT_CONFIG":T11)  [unwired: 1 out]
        n163 = Bundle("ID"="ID", w176, w175, "发送类型"="发送类型", "帧格式"="帧格式", "帧类型"="帧类型", w172, "[0]"=w180, "[1]"=w181, "[2]"=w182, "[3]"=w183, "[4]"=w184, "[5]"=w185, "[6]"=w186, "[7]"=w187, w188, w188, w188) -> (w190:T12)  [unwired: 1 out]
        n164 = local write "VCI_CAN_OBJ_T"(w190) -> ()
        n165 = local read "寄存器"() -> (w153:u32)
        n166 = Bundle("寄存器"=w153) -> (w158:cluster{"寄存器":u32})  [unwired: 1 in]
        n167 = local write "e-u-baud"(w158) -> ()
      }
      event "DBC发送界面": Value Change {
        n168 = event-data() -> ()  [unwired: 7 out]
        n169 = flat-sequence {
          frame #0 {
            n170 = local write "DBC界面"(TRUE ("DBC界面")) -> ()
          }
          frame #1 {
            w216 = u16 0 items=["ControlCAN", "zlgcan"]
            n171 = local read "CANStartup"() -> (w212:bool)
            n172 = local read "CAN 通道"() -> (w213:u32)
            n173 = local read "设备类型"() -> (w215:u32)
            n174 = local read "索引"() -> (w214:u32)
            n175 = call "dbc_demo.vi"("DLL类型"=w216, "设备类型"=w215, "设备索引"=w214, "通道索引"=w213, "设备打开状态"=w212) -> ()  [unwired: 11 in]
          }
          frame #2 {
            n176 = local write "DBC界面"(FALSE ("DBC界面")) -> ()
          }
        }
      }
      event "定时发送": Value Change {
        w218 = u8 0
        n177 = event-data() -> ()  [unwired: 7 out]
        n178 = local read "VCI_CAN_OBJ_T"() -> (w219:T6)
        n179 = local read "设备类型值"() -> (w232:u32)
        n180 = local read "CAN 通道"() -> (w233:u32)
        n181 = local read "索引"() -> (w230:u32)
        n182 = Bundle(u8 1, u8 1, w218, w218, u32 1000, "VCI_CAN_OBJ_T"=w219) -> (w225:T13)  [unwired: 1 in]
        n183 = dll-call lib="E:/Project/CANMaster/LabView/ControlCAN_labview/bin/ControlCAN.dll" fn="VCI_SetReference"("DevType"=w232, "DevIndex"=w230, "CANInd"=w233, "RefType"=u32 5, "pData"=w225) -> ("返回类型"=w231:u32)  [unwired: 7 in, 3 out]
        n184 = Equal?(x=w231, y=u32 1) -> (x = y?=w224:bool)
        n185 = Select(t="定时发送设置成功。", s=w224, f="定时发送设置失败！") -> (s? t:f=w221:string)
        n186 = One Button Dialog(message=w221) -> ()  [unwired: 1 in, 1 out]
      }
      event "清除定时发送": Value Change {
        n187 = event-data() -> ()  [unwired: 7 out]
        n188 = local read "设备类型值"() -> (w244:u32)
        n189 = local read "CAN 通道"() -> (w245:u32)
        n190 = local read "索引"() -> (w242:u32)
        n191 = Bundle(0) -> (w234:cluster{i32})  [unwired: 1 in]
        n192 = dll-call lib="E:/Project/CANMaster/LabView/ControlCAN_labview/bin/ControlCAN.dll" fn="VCI_SetReference"("DevType"=w244, "DevIndex"=w242, "CANInd"=w245, "RefType"=u32 6, "pData"=w234) -> ("返回类型"=w243:u32)  [unwired: 7 in, 3 out]
        n193 = Equal?(x=w243, y=u32 1) -> (x = y?=w241:bool)
        n194 = Select(t="清除定时发送成功。", s=w241, f="清除定时发送失败！") -> (s? t:f=w240:string)
        n195 = One Button Dialog(message=w240) -> ()  [unwired: 1 in, 1 out]
      }
      event "Baud": Value Change {
        n196 = event-data() -> ()  [unwired: 7 out]
        n197 = local read "Baud"() -> (w246:u32)
        n198 = case shown="15, 默认" w246 {
          frame 0 {
            n199 = local write "BTR0"(u8 191 ("BTR0")) -> ()
            n200 = local write "BTR1"(u8 255 ("BTR1")) -> ()
          }
          frame 1 {
            n201 = local write "BTR0"(49) -> ()
            n202 = local write "BTR1"(28) -> ()
          }
          frame 2 {
            n203 = local write "BTR0"(24) -> ()
            n204 = local write "BTR1"(28) -> ()
          }
          frame 3 {
            n205 = local write "BTR0"(135) -> ()
            n206 = local write "BTR1"(255) -> ()
          }
          frame 4 {
            n207 = local write "BTR0"(9) -> ()
            n208 = local write "BTR1"(28) -> ()
          }
          frame 5 {
            n209 = local write "BTR1"(255) -> ()
            n210 = local write "BTR0"(131) -> ()
          }
          frame 6 {
            n211 = local write "BTR1"(28) -> ()
            n212 = local write "BTR0"(4) -> ()
          }
          frame 7 {
            n213 = local write "BTR1"(28) -> ()
            n214 = local write "BTR0"(3) -> ()
          }
          frame 8 {
            n215 = local write "BTR0"(129) -> ()
            n216 = local write "BTR1"(250) -> ()
          }
          frame 9 {
            n217 = local write "BTR0"(1) -> ()
            n218 = local write "BTR1"(28) -> ()
          }
          frame 10 {
            n219 = local write "BTR1"(250) -> ()
            n220 = local write "BTR0"(128) -> ()
          }
          frame 11 {
            n221 = local write "BTR0"(0) -> ()
            n222 = local write "BTR1"(28) -> ()
          }
          frame 12 {
            n223 = local write "BTR1"(182) -> ()
            n224 = local write "BTR0"(128) -> ()
          }
          frame 13 {
            n225 = local write "BTR0"(0) -> ()
            n226 = local write "BTR1"(22) -> ()
          }
          frame 14 {
            n227 = local write "BTR0"(0) -> ()
            n228 = local write "BTR1"(20) -> ()
          }
          frame 15, Default {
            n229 = local write "BTR0"(1) -> ()
            n230 = local write "BTR1"(1) -> ()
          }
        }
      }
      event "Radio_Baud": Value Change {
        n231 = event-data() -> ()  [unwired: 7 out]
        n232 = local read "Radio_Baud"() -> (w279:bool)
        n233 = case shown="假" w279 {
          frame False {
            n234 = property on="BTR1" class="DigNum (严格)"("Disabled"=2) -> ()  [unwired: 2 in, 2 out]
            n235 = property on="BTR0" class="DigNum (严格)"("Disabled"=2) -> ()  [unwired: 2 in, 2 out]
            n236 = property on="Baud" class="Ring (严格)"("Disabled"=0) -> ()  [unwired: 2 in, 2 out]
          }
          frame True {
            n237 = property on="BTR0" class="DigNum (严格)"("Disabled"=0) -> ()  [unwired: 2 in, 2 out]
            n238 = property on="BTR1" class="DigNum (严格)"("Disabled"=0) -> ()  [unwired: 2 in, 2 out]
            n239 = property on="Baud" class="Ring (严格)"("Disabled"=2) -> ()  [unwired: 2 in, 2 out]
          }
        }
      }
      event "stop": Value Change {
        n240 = event-data() -> ()  [unwired: 2 out]
        n241 = stacked-sequence {
          tunnel: [_ _ "stop"] -> w286
          frame #0 {
            n242 = local read "DeviceOpen"() -> (w287:bool)
            n243 = case shown="真" w287 {
              frame False {
              }
              frame True {
                w288 = u8 0 ("Disabled")
                n244 = local read "设备类型值"() -> (w290:u32)
                n245 = property on="设备类型值" class="Ring (严格)"("禁用"=w288) -> ()  [unwired: 2 in, 2 out]
                n246 = property on="CAN 通道" class="Ring (严格)"("禁用"=w288) -> ()  [unwired: 2 in, 2 out]
                n247 = property on="索引" class="Ring (严格)"("Disabled"=w288) -> ()  [unwired: 2 in, 2 out]
                n248 = dll-call lib="E:/Project/CANMaster/LabView/ControlCAN_labview/bin/ControlCAN.dll" fn="VCI_CloseDevice"("DeviceType"=w290, "DeviceInd"=0) -> (w292:u32)  [unwired: 5 in, 2 out]
                n249 = Equal?(x=w292, y=u32 1) -> (x = y?=w289:bool)
                n250 = case shown="真" w289 {
                  frame False {
                  }
                  frame True {
                    w294 = u8 0 ("禁用")
                    w295 = u8 0 ("Disabled")
                    w297 = FALSE ("DeviceOpen")
                    n251 = property on="OpenDevice" class="Bool"("布尔文本.文本"="打开设备" ("Boolean Text.Text")) -> ()  [unwired: 2 in, 2 out]
                    n252 = local write "DeviceOpen"(w297) -> ()
                    n253 = local write "CANStartup"(w297) -> ()
                    n254 = property on="验收码" class="DigNum (严格)"("禁用"=w295) -> ()  [unwired: 2 in, 2 out]
                    n255 = property on="屏蔽码" class="DigNum (严格)"("禁用"=w295) -> ()  [unwired: 2 in, 2 out]
                    n256 = property on="滤波方式" class="Ring (严格)"("禁用"=w295) -> ()  [unwired: 2 in, 2 out]
                    n257 = property on="BTR0" class="DigNum (严格)"("禁用"=w295) -> ()  [unwired: 2 in, 2 out]
                    n258 = property on="BTR1" class="DigNum (严格)"("禁用"=w295) -> ()  [unwired: 2 in, 2 out]
                    n259 = property on="模式" class="Ring (严格)"("禁用"=w295) -> ()  [unwired: 2 in, 2 out]
                    n260 = property on="Baud(E_U)" class="Ring (严格)"("Disabled"=w294) -> ()  [unwired: 2 in, 2 out]
                    n261 = property on="滤波起始ID" class="DigNum (严格)"("Disabled"=w294) -> ()  [unwired: 2 in, 2 out]
                    n262 = property on="滤波模式" class="Ring (严格)"("Disabled"=w294) -> ()  [unwired: 2 in, 2 out]
                    n263 = property on="滤波结束ID" class="DigNum (严格)"("Disabled"=w294) -> ()  [unwired: 2 in, 2 out]
                  }
                }
              }
            }
          }
          frame #1 {
            n264 = Wait Until Next ms Multiple(millisecond multiple=u32 500) -> ()  [unwired: 1 out]
            "stop 2" <- TRUE ("stop 2")
          }
          frame #2 {
          }
        }
      }
      event "OpenDevice": Value Change {
        n265 = event-data() -> ()  [unwired: 2 out]
        n266 = case shown="真" "DeviceOpen" {
          frame False {
            w307 = u32 12 items=["PCI5121"=1, "PCI9810"=2, "USBCAN1"=3, "USBCAN2"=4, "PCI9820"=5, "PCI5110"=7, "CANLite(mini)"=8, "ISA9620"=9, "ISA5420"=10, "PC104CAN"=11, "CANETUDP"=12, "DNP9810"=13, "PCI9840B"=14, "PC104C2"=15, "PCI9820I"=16, "CANETTCP"=17, "pec9920"=18, "PCI5010U"=19, "USBCAN_E_U"=20, "USBCAN_2E_U"=21, "PCI5020U"=22] ("DeviceType")
            # "判断使用canet udp模式"
            n267 = local read "设备类型值"() -> (w312:u32)
            n268 = local read "设备类型值"() -> (w308:u32)
            n269 = local read "本机端口"() -> (w306:u32)
            n270 = Equal?(x=w308, y=w307) -> (x = y?=w302:bool)
            n271 = Select(t=w306, s=w302, f=u32 0) -> (s? t:f=w304:u32)
            n272 = dll-call lib="E:/Project/CANMaster/LabView/ControlCAN_labview/bin/ControlCAN.dll" fn="VCI_OpenDevice"("DevType"=w312, "DevIndex"=0, "Reserved"=w304) -> (w311:u32)  [unwired: 6 in, 2 out]
            n273 = Equal?(x=w311, y=u32 1) -> (x = y?=w309:bool)
            n274 = case shown="真" w309 {
              frame False {
                n275 = call "显示对话框信息7"() -> ()  [unwired: 3 in, 9 out]
              }
              frame True {
                n276 = stacked-sequence {
                  seq-local: [w313 _ _ _ _ _ _] -> [_ w326 _ w373 _ _ _]
                  frame #0 {
                    w318 = u32 19 items=["PCI5121"=1, "PCI9810"=2, "USBCAN1"=3, "USBCAN2"=4, "PCI9820"=5, "PCI5110"=7, "CANLite(mini)"=8, "ISA9620"=9, "ISA5420"=10, "PC104CAN"=11, "DNP9810"=13, "PCI9840B"=14, "PC104C2"=15, "PCI9820I"=16, "pec9920"=18, "PCI5010U"=19, "USBCAN_E_U"=20, "USBCAN_2E_U"=21, "PCI5020U"=22, ""=0] ("DeviceType")
                    w320 = u32 22 items=["PCI5121"=1, "PCI9810"=2, "USBCAN1"=3, "USBCAN2"=4, "PCI9820"=5, "PCI5110"=7, "CANLite(mini)"=8, "ISA9620"=9, "ISA5420"=10, "PC104CAN"=11, "DNP9810"=13, "PCI9840B"=14, "PC104C2"=15, "PCI9820I"=16, "pec9920"=18, "PCI5010U"=19, "USBCAN_E_U"=20, "USBCAN_2E_U"=21, "PCI5020U"=22, ""=0] ("DeviceType")
                    w324 = u32 21 items=["PCI5121"=1, "PCI9810"=2, "USBCAN1"=3, "USBCAN2"=4, "PCI9820"=5, "PCI5110"=7, "CANLite(mini)"=8, "ISA9620"=9, "ISA5420"=10, "PC104CAN"=11, "DNP9810"=13, "PCI9840B"=14, "PC104C2"=15, "PCI9820I"=16, "pec9920"=18, "USBCAN_E_U"=20, "USBCAN_2E_U"=21, ""=0] ("DeviceType")
                    w325 = u32 20 items=["PCI5121"=1, "PCI9810"=2, "USBCAN1"=3, "USBCAN2"=4, "PCI9820"=5, "PCI5110"=7, "CANLite(mini)"=8, "ISA9620"=9, "ISA5420"=10, "PC104CAN"=11, "DNP9810"=13, "PCI9840B"=14, "PC104C2"=15, "PCI9820I"=16, "pec9920"=18, "USBCAN_E_U"=20, "USBCAN_2E_U"=21, ""=0] ("DeviceType")
                    # "判断是不是USB_U_E设备"
                    n277 = local read "设备类型值"() -> (w319:u32)
                    n278 = Equal?(x=w319, y=w325) -> (x = y?=w323:bool)
                    n279 = Equal?(x=w319, y=w324) -> (x = y?=w322:bool)
                    n280 = Equal?(x=w319, y=w320) -> (x = y?=w317:bool)
                    n281 = Equal?(x=w319, y=w318) -> (x = y?=w316:bool)
                    n282 = Or(x=w323, y=w322) -> (x .or. y?=w315:bool)
                    n283 = Or(x=w317, y=w316) -> (x .or. y?=w314:bool)
                    n284 = Or(x=w315, y=w314) -> (x .or. y?=w313:bool)
                    n285 = global write "globe.vi" "ret_ok"(TRUE ("ret_ok")) -> ()
                  }
                  frame #1 {
                    n286 = case shown="真" w326 {
                      frame False {
                        # "不是 -U-E 设备"
                        n287 = local read "Baud"() -> (w328:u32)
                        n288 = case shown="0, 默认" w328 {
                          tunnel: [5120 10240 20480 40960 51200 81920 102400 128000 204800 256000 409600 512000 681984 819200 1024000] -> w327
                          frame 0, Default {
                          }
                          frame 1 {
                          }
                          frame 2 {
                          }
                          frame 3 {
                          }
                          frame 4 {
                          }
                          frame 5 {
                          }
                          frame 6 {
                          }
                          frame 7 {
                          }
                          frame 8 {
                          }
                          frame 9 {
                          }
                          frame 10 {
                          }
                          frame 11 {
                          }
                          frame 12 {
                          }
                          frame 13 {
                          }
                          frame 14 {
                          }
                        }
                        n289 = global write "globe.vi" "通道波特率"(w327) -> ()
                      }
                      frame True {
                        # "设置波特率"
                        # "USB-E-U初始化"
                        n290 = local read "设备类型值"() -> (w353:u32)
                        n291 = local read "CAN 通道"() -> (w347:u32)
                        n292 = local read "索引"() -> (w348:u32)
                        n293 = local read "e-u-baud"() -> (w349:cluster{"数值":u32})
                        n294 = local read "Baud(E_U)"() -> (w345:u32)
                        n295 = dll-call lib="E:/Project/CANMaster/LabView/ControlCAN_labview/bin/ControlCAN.dll" fn="VCI_SetReference"("DevType"=w353, "DevIndex"=w348, "CANInd"=w347, "RefType"=u32 0 ("y"), "pData"=w349) -> ("返回类型"=w352:u32)  [unwired: 8 in, 2 out]
                        n296 = case shown="60003, 默认" w345 {
                          tunnel: [1024000 819200 512000 256000 128000 102400 51200 20480 10240 5120] -> w344
                          frame 393219, Default {
                          }
                          frame 393220 {
                          }
                          frame 393223 {
                          }
                          frame 1835016 {
                          }
                          frame 1835025 {
                          }
                          frame 1441827 {
                          }
                          frame 1835052 {
                          }
                          frame 1441971 {
                          }
                          frame 1835232 {
                          }
                          frame 1835457 {
                          }
                        }
                        n297 = Equal?(x=w352, y=u32 1) -> (x = y?=w350:bool)
                        n298 = global write "globe.vi" "通道波特率"(w344) -> ()
                        n299 = case shown="假" w350 {
                          frame False {
                            n300 = call "显示对话框信息3"() -> ()  [unwired: 3 in, 9 out]
                          }
                          frame True {
                          }
                        }
                        n301 = global write "globe.vi" "ret_ok"(w350) -> ()
                      }
                    }
                  }
                  frame #2 {
                    n302 = global read "globe.vi" "ret_ok"() -> (w364:bool)
                    n303 = case shown="真" w364 {
                      frame False {
                      }
                      frame True {
                        n304 = local read "CAN 通道"() -> (w371:u32)
                        n305 = local read "索引"() -> (w365:u32)
                        n306 = local read "设备类型值"() -> (w370:u32)
                        n307 = local read "VCI_INIT_CONFIG"() -> (w369:T7)
                        n308 = dll-call lib="E:/Project/CANMaster/LabView/ControlCAN_labview/bin/ControlCAN.dll" fn="VCI_InitCAN"("DeviceType"=w370, "DeviceInd"=w365, "CANInd"=w371, "VCI_INIT_CONFIG"=w369) -> (w368:u32)  [unwired: 7 in, 2 out]
                        n309 = Equal?(x=w368, y=u32 1) -> (x = y?=w366:bool)
                        n310 = case shown="假" w366 {
                          frame False {
                            n311 = call "显示对话框信息6"() -> ()  [unwired: 3 in, 9 out]
                          }
                          frame True {
                          }
                        }
                        n312 = global write "globe.vi" "ret_ok"(w366) -> ()
                      }
                    }
                  }
                  frame #3 {
                    n313 = global read "globe.vi" "ret_ok"() -> (w372:bool)
                    n314 = And(x=w373, y=w372) -> (x .and. y?=w374:bool)
                    n315 = case shown="真" w374 {
                      frame False {
                      }
                      frame True {
                        w377 = u32 2 items=["标准帧滤波", "扩展帧滤波", "禁能滤波"] ("fiter_mode")
                        # "设置波特率正确，就设置滤波"
                        n316 = local read "滤波模式"() -> (w376:u32)
                        n317 = Not Equal?(x=w376, y=w377) -> (x != y?=w375:bool)
                        n318 = case shown="真" w375 {
                          frame False {
                          }
                          frame True {
                            n319 = stacked-sequence {
                              frame #0 {
                                n320 = local read "VCI_FILTER_RECORD"() -> (w379:cluster{"ExtFrame":u32, "Start":u32, "End":u32})
                                n321 = local read "设备类型值"() -> (w381:u32)
                                n322 = local read "CAN 通道"() -> (w382:u32)
                                n323 = local read "索引"() -> (w378:u32)
                                n324 = dll-call lib="E:/Project/CANMaster/LabView/ControlCAN_labview/bin/ControlCAN.dll" fn="VCI_SetReference"("DevType"=w381, "DevIndex"=w378, "CANInd"=w382, "RefType"=u32 1, "pData"=w379) -> ()  [unwired: 8 in, 3 out]
                              }
                              frame #1 {
                                n325 = local read "设备类型值"() -> (w389:u32)
                                n326 = local read "CAN 通道"() -> (w390:u32)
                                n327 = local read "索引"() -> (w383:u32)
                                n328 = dll-call lib="E:/Project/CANMaster/LabView/ControlCAN_labview/bin/ControlCAN.dll" fn="VCI_SetReference"("DevType"=w389, "DevIndex"=w383, "CANInd"=w390, "RefType"=u32 2, "pData"=u32 0 ("RefType")) -> ("返回类型"=w386:u32)  [unwired: 7 in, 3 out]
                                n329 = Equal?(x=w386, y=u32 1) -> (x = y?=w384:bool)
                                n330 = case shown="假" w384 {
                                frame False {
                                n331 = call "显示对话框信息4"() -> ()  [unwired: 3 in, 9 out]
                                }
                                frame True {
                                }
                                }
                                n332 = global write "globe.vi" "ret_ok"(w384) -> ()
                              }
                            }
                          }
                        }
                      }
                    }
                  }
                  frame #4 {
                    w399 = u32 17 items=["PCI5121"=1, "PCI9810"=2, "USBCAN1"=3, "USBCAN2"=4, "PCI9820"=5, "PCI5110"=7, "CANLite(mini)"=8, "ISA9620"=9, "ISA5420"=10, "PC104CAN"=11, "CANETUDP"=12, "DNP9810"=13, "PCI9840B"=14, "PC104C2"=15, "PCI9820I"=16, "CANETTCP"=17, "pec9920"=18, "PCI5010U"=19, "USBCAN_E_U"=20, "USBCAN_2E_U"=21, "PCI5020U"=22] ("DeviceType")
                    w400 = u32 12 items=["PCI5121"=1, "PCI9810"=2, "USBCAN1"=3, "USBCAN2"=4, "PCI9820"=5, "PCI5110"=7, "CANLite(mini)"=8, "ISA9620"=9, "ISA5420"=10, "PC104CAN"=11, "CANETUDP"=12, "DNP9810"=13, "PCI9840B"=14, "PC104C2"=15, "PCI9820I"=16, "CANETTCP"=17, "pec9920"=18, "PCI5010U"=19, "USBCAN_E_U"=20, "USBCAN_2E_U"=21, "PCI5020U"=22] ("DeviceType")
                    # "如果是UDP模式 或者是 TCP客户端模式"
                    # "客户端模式"
                    # "canet tcp模式"
                    # "判断使用canet udp模式"
                    n333 = local read "本机类型"() -> (w397:enum32{"Radio Selection 1", "Radio Selection 2"})
                    n334 = local read "设备类型值"() -> (w398:u32)
                    n335 = Equal?(x=w398, y=w399) -> (x = y?=w394:bool)
                    n336 = Equal?(x=enum32{"Radio Selection 1", "Radio Selection 2"}."Radio Selection 2", y=w397) -> (x = y?=w395:bool)
                    n337 = Equal?(x=w398, y=w400) -> (x = y?=w393:bool)
                    n338 = And(x=w394, y=w395) -> (x .and. y?=w392:bool)
                    n339 = Or(x=w393, y=w392) -> (x .or. y?=w391:bool)
                    n340 = case shown="真" w391 {
                      frame False {
                      }
                      frame True {
                        n341 = stacked-sequence {
                          frame #0 {
                            # "1 端口命令"
                            # "设置 端口"
                            n342 = local read "CANET 端口"() -> (w404:u32)
                            n343 = local read "设备类型值"() -> (w408:u32)
                            n344 = local read "CAN 通道"() -> (w409:u32)
                            n345 = local read "索引"() -> (w401:u32)
                            n346 = call "LongToByteArr.vi"("CANET 端口"=w404) -> ("Array"=w403:u8[])
                            n347 = dll-call lib="E:/Project/CANMaster/LabView/ControlCAN_labview/bin/ControlCAN.dll" fn="VCI_SetReference"("DevType"=w408, "DevIndex"=w401, "CANInd"=w409, "RefType"=u32 1, "pData"=w403) -> ("返回类型"=w405:u32)  [unwired: 8 in, 2 out]
                            n348 = Equal?(x=w405, y=u32 1) -> (x = y?=w402:bool)
                            n349 = case shown="假" w402 {
                              frame False {
                                n350 = call "显示对话框信息11"() -> ()  [unwired: 3 in, 9 out]
                              }
                              frame True {
                              }
                            }
                            n351 = global write "globe.vi" "ret_ok"(w402) -> ()
                          }
                          frame #1 {
                            # "0 ip命令"
                            # "设置CANET ip"
                            n352 = local read "CANET IP"() -> (w415:string)
                            n353 = local read "设备类型值"() -> (w420:u32)
                            n354 = local read "CAN 通道"() -> (w421:u32)
                            n355 = local read "索引"() -> (w410:u32)
                            n356 = String To Byte Array(string=w415) -> (unsigned byte array=w413:u8[])
                            n357 = Array Size(array=w413) -> (size(s)=w414:i32)
                            n358 = Insert Into Array(array=w413, index=w414, new element=u8 0 ("new element/subarray")) -> (w411:u8[])
                            n359 = dll-call lib="E:/Project/CANMaster/LabView/ControlCAN_labview/bin/ControlCAN.dll" fn="VCI_SetReference"("DevType"=w420, "DevIndex"=w410, "CANInd"=w421, "RefType"=u32 0, "pData"=w411) -> ("返回类型"=w418:u32)  [unwired: 8 in, 2 out]
                            n360 = Equal?(x=w418, y=u32 1) -> (x = y?=w416:bool)
                            n361 = global write "globe.vi" "ret_ok"(w416) -> ()
                            n362 = case shown="假" w416 {
                              frame False {
                                n363 = call "显示对话框信息8"() -> ()  [unwired: 3 in, 9 out]
                              }
                              frame True {
                              }
                            }
                          }
                          frame #2 {
                            w423 = u8 0 ("element")
                            # "设置 客户端模式"
                            # "0 模式命令"
                            n364 = local read "设备类型值"() -> (w428:u32)
                            n365 = local read "CAN 通道"() -> (w429:u32)
                            n366 = local read "索引"() -> (w422:u32)
                            n367 = Build Array(w423, w423, w423, w423) -> (w424:u8[])
                            n368 = dll-call lib="E:/Project/CANMaster/LabView/ControlCAN_labview/bin/ControlCAN.dll" fn="VCI_SetReference"("DevType"=w428, "DevIndex"=w422, "CANInd"=w429, "RefType"=u32 4, "pData"=w424) -> ("返回类型"=w427:u32)  [unwired: 7 in, 3 out]
                            n369 = Equal?(x=w427, y=u32 1) -> ()  [unwired: 1 out]
                          }
                        }
                      }
                    }
                  }
                  frame #5 {
                    w436 = u32 17 items=["PCI5121"=1, "PCI9810"=2, "USBCAN1"=3, "USBCAN2"=4, "PCI9820"=5, "PCI5110"=7, "CANLite(mini)"=8, "ISA9620"=9, "ISA5420"=10, "PC104CAN"=11, "CANETUDP"=12, "DNP9810"=13, "PCI9840B"=14, "PC104C2"=15, "PCI9820I"=16, "CANETTCP"=17, "pec9920"=18, "PCI5010U"=19, "USBCAN_E_U"=20, "USBCAN_2E_U"=21, "PCI5020U"=22] ("DeviceType")
                    # "服务器模式"
                    # "canet tcp模式"
                    n370 = local read "设备类型值"() -> (w431:u32)
                    n371 = local read "本机类型"() -> (w435:enum32{"Radio Selection 1", "Radio Selection 2"})
                    n372 = Equal?(x=w431, y=w436) -> (x = y?=w432:bool)
                    n373 = Equal?(x=enum32{"Radio Selection 1", "Radio Selection 2"}."Radio Selection 1", y=w435) -> (x = y?=w433:bool)
                    n374 = And(x=w432, y=w433) -> (x .and. y?=w430:bool)
                    n375 = case shown="真" w430 {
                      frame False {
                      }
                      frame True {
                        # "如果是 tcp 服务器模式"
                        n376 = stacked-sequence {
                          frame #0 {
                            # "2 本机端口命令"
                            # "设置 服务器 本机端口"
                            n377 = local read "本机端口"() -> (w439:u32)
                            n378 = local read "设备类型值"() -> (w444:u32)
                            n379 = local read "CAN 通道"() -> (w445:u32)
                            n380 = local read "索引"() -> (w437:u32)
                            n381 = call "LongToByteArr.vi"("CANET 端口"=w439) -> ("Array"=w438:u8[])
                            n382 = dll-call lib="E:/Project/CANMaster/LabView/ControlCAN_labview/bin/ControlCAN.dll" fn="VCI_SetReference"("DevType"=w444, "DevIndex"=w437, "CANInd"=w445, "RefType"=u32 2, "pData"=w438) -> ("返回类型"=w441:u32)  [unwired: 8 in, 2 out]
                            n383 = Equal?(x=w441, y=u32 1) -> (x = y?=w440:bool)
                            n384 = case shown="假" w440 {
                              frame False {
                                n385 = call "显示对话框信息10"() -> ()  [unwired: 3 in, 9 out]
                              }
                              frame True {
                              }
                            }
                            n386 = global write "globe.vi" "ret_ok"(w440) -> ()
                          }
                          frame #1 {
                            # "0 模式命令"
                            # "设置 服务器模式"
                            n387 = local read "设备类型值"() -> (w452:u32)
                            n388 = local read "CAN 通道"() -> (w453:u32)
                            n389 = local read "索引"() -> (w446:u32)
                            n390 = local read "type"() -> (w447:u8[])
                            n391 = dll-call lib="E:/Project/CANMaster/LabView/ControlCAN_labview/bin/ControlCAN.dll" fn="VCI_SetReference"("DevType"=w452, "DevIndex"=w446, "CANInd"=w453, "RefType"=u32 4, "pData"=w447) -> ("返回类型"=w450:u32)  [unwired: 8 in, 2 out]
                            n392 = Equal?(x=w450, y=u32 1) -> (x = y?=w448:bool)
                            n393 = case shown="假" w448 {
                              frame False {
                                n394 = call "显示对话框信息9"() -> ()  [unwired: 3 in, 9 out]
                              }
                              frame True {
                              }
                            }
                            n395 = global write "globe.vi" "ret_ok"(w448) -> ()
                          }
                        }
                      }
                    }
                  }
                  frame #6 {
                    n396 = global read "globe.vi" "ret_ok"() -> (w454:bool)
                    n397 = case shown="真" w454 {
                      frame False {
                        n398 = local read "设备类型值"() -> (w456:u32)
                        n399 = local read "索引"() -> (w455:u32)
                        n400 = dll-call lib="E:/Project/CANMaster/LabView/ControlCAN_labview/bin/ControlCAN.dll" fn="VCI_CloseDevice"("DeviceType"=w456, "DeviceInd"=w455) -> ()  [unwired: 5 in, 3 out]
                        n401 = call "显示对话框信息5"() -> ()  [unwired: 3 in, 9 out]
                      }
                      frame True {
                        w457 = u8 2 ("Disabled")
                        w461 = u8 2 ("禁用")
                        n402 = property on="OpenDevice" class="Bool"("布尔文本.文本"="关闭设备") -> ()  [unwired: 2 in, 2 out]
                        n403 = property on="设备类型值" class="Ring (严格)"("禁用"=u8 2 ("Disabled")) -> ()  [unwired: 2 in, 2 out]
                        n404 = local write "DeviceOpen"(TRUE ("DeviceOpen")) -> ()
                        n405 = property on="Radio_Baud" class="Bool (严格)"("Disabled"=w457) -> ()  [unwired: 2 in, 2 out]
                        n406 = property on="验收码" class="DigNum (严格)"("禁用"=w457) -> ()  [unwired: 2 in, 2 out]
                        n407 = property on="屏蔽码" class="DigNum (严格)"("禁用"=w457) -> ()  [unwired: 2 in, 2 out]
                        n408 = property on="滤波方式" class="Ring (严格)"("禁用"=w457) -> ()  [unwired: 2 in, 2 out]
                        n409 = property on="Baud" class="Ring (严格)"("Disabled"=w457) -> ()  [unwired: 2 in, 2 out]
                        n410 = property on="BTR0" class="DigNum (严格)"("禁用"=w457) -> ()  [unwired: 2 in, 2 out]
                        n411 = property on="BTR1" class="DigNum (严格)"("禁用"=w457) -> ()  [unwired: 2 in, 2 out]
                        n412 = property on="模式" class="Ring (严格)"("禁用"=w457) -> ()  [unwired: 2 in, 2 out]
                        n413 = property on="Baud(E_U)" class="Ring (严格)"("Disabled"=w461) -> ()  [unwired: 2 in, 2 out]
                        n414 = property on="滤波起始ID" class="DigNum (严格)"("Disabled"=w461) -> ()  [unwired: 2 in, 2 out]
                        n415 = property on="滤波模式" class="Ring (严格)"("Disabled"=w461) -> ()  [unwired: 2 in, 2 out]
                        n416 = property on="滤波结束ID" class="DigNum (严格)"("Disabled"=w461) -> ()  [unwired: 2 in, 2 out]
                      }
                    }
                  }
                }
              }
            }
          }
          frame True {
            n417 = stacked-sequence {
              frame #0 {
                n418 = local read "设备类型值"() -> (w465:u32)
                n419 = dll-call lib="E:/Project/CANMaster/LabView/ControlCAN_labview/bin/ControlCAN.dll" fn="VCI_CloseDevice"("DeviceType"=w465, "DeviceInd"=0) -> (w464:u32)  [unwired: 5 in, 2 out]
                n420 = Equal?(x=w464, y=u32 1) -> (x = y?=w462:bool)
                n421 = case shown="真" w462 {
                  frame False {
                  }
                  frame True {
                    w468 = u8 0 ("禁用")
                    w469 = u8 0 ("Disabled")
                    w467 = u8 0 ("Disabled")
                    w471 = FALSE
                    n422 = property on="OpenDevice" class="Bool"("布尔文本.文本"="打开设备" ("Boolean Text.Text")) -> ()  [unwired: 2 in, 2 out]
                    n423 = property on="CAN 通道" class="Ring (严格)"("禁用"=w467) -> ()  [unwired: 2 in, 2 out]
                    n424 = property on="设备类型值" class="Ring (严格)"("禁用"=w467) -> ()  [unwired: 2 in, 2 out]
                    n425 = local write "CANStartup"(w471) -> ()
                    n426 = local write "DeviceOpen"(w471) -> ()
                    n427 = property on="索引" class="Ring (严格)"("Disabled"=w467) -> ()  [unwired: 2 in, 2 out]
                    n428 = property on="验收码" class="DigNum (严格)"("禁用"=w469) -> ()  [unwired: 2 in, 2 out]
                    n429 = property on="屏蔽码" class="DigNum (严格)"("禁用"=w469) -> ()  [unwired: 2 in, 2 out]
                    n430 = property on="滤波方式" class="Ring (严格)"("禁用"=w469) -> ()  [unwired: 2 in, 2 out]
                    n431 = property on="BTR0" class="DigNum (严格)"("禁用"=w469) -> ()  [unwired: 2 in, 2 out]
                    n432 = property on="BTR1" class="DigNum (严格)"("禁用"=w469) -> ()  [unwired: 2 in, 2 out]
                    n433 = property on="模式" class="Ring (严格)"("禁用"=w469) -> ()  [unwired: 2 in, 2 out]
                    n434 = property on="Baud(E_U)" class="Ring (严格)"("Disabled"=w468) -> ()  [unwired: 2 in, 2 out]
                    n435 = property on="滤波起始ID" class="DigNum (严格)"("Disabled"=w468) -> ()  [unwired: 2 in, 2 out]
                    n436 = property on="滤波模式" class="Ring (严格)"("Disabled"=w468) -> ()  [unwired: 2 in, 2 out]
                    n437 = property on="滤波结束ID" class="DigNum (严格)"("Disabled"=w468) -> ()  [unwired: 2 in, 2 out]
                  }
                }
              }
              frame #1 {
                w480 = u32 19 items=["PCI5121"=1, "PCI9810"=2, "USBCAN1"=3, "USBCAN2"=4, "PCI9820"=5, "PCI5110"=7, "CANLite(mini)"=8, "ISA9620"=9, "ISA5420"=10, "PC104CAN"=11, "DNP9810"=13, "PCI9840B"=14, "PC104C2"=15, "PCI9820I"=16, "pec9920"=18, "PCI5010U"=19, "USBCAN_E_U"=20, "USBCAN_2E_U"=21, "PCI5020U"=22, ""=0] ("DeviceType")
                w481 = u32 22 items=["PCI5121"=1, "PCI9810"=2, "USBCAN1"=3, "USBCAN2"=4, "PCI9820"=5, "PCI5110"=7, "CANLite(mini)"=8, "ISA9620"=9, "ISA5420"=10, "PC104CAN"=11, "DNP9810"=13, "PCI9840B"=14, "PC104C2"=15, "PCI9820I"=16, "pec9920"=18, "PCI5010U"=19, "USBCAN_E_U"=20, "USBCAN_2E_U"=21, "PCI5020U"=22, ""=0] ("DeviceType")
                w482 = u32 21 items=["PCI5121"=1, "PCI9810"=2, "USBCAN1"=3, "USBCAN2"=4, "PCI9820"=5, "PCI5110"=7, "CANLite(mini)"=8, "ISA9620"=9, "ISA5420"=10, "PC104CAN"=11, "DNP9810"=13, "PCI9840B"=14, "PC104C2"=15, "PCI9820I"=16, "pec9920"=18, "USBCAN_E_U"=20, "USBCAN_2E_U"=21, ""=0] ("DeviceType")
                w483 = u32 20 items=["PCI5121"=1, "PCI9810"=2, "USBCAN1"=3, "USBCAN2"=4, "PCI9820"=5, "PCI5110"=7, "CANLite(mini)"=8, "ISA9620"=9, "ISA5420"=10, "PC104CAN"=11, "DNP9810"=13, "PCI9840B"=14, "PC104C2"=15, "PCI9820I"=16, "pec9920"=18, "USBCAN_E_U"=20, "USBCAN_2E_U"=21, ""=0] ("DeviceType")
                n438 = local read "设备类型值"() -> (w479:u32)
                n439 = Equal?(x=w479, y=w483) -> (x = y?=w478:bool)
                n440 = Equal?(x=w479, y=w482) -> (x = y?=w477:bool)
                n441 = Equal?(x=w479, y=w481) -> (x = y?=w476:bool)
                n442 = Equal?(x=w479, y=w480) -> (x = y?=w475:bool)
                n443 = Or(x=w476, y=w475) -> (x .or. y?=w473:bool)
                n444 = Or(x=w478, y=w477) -> (x .or. y?=w474:bool)
                n445 = Or(x=w474, y=w473) -> (x .or. y?=w472:bool)
                n446 = case shown="真" w472 {
                  frame False {
                    n447 = stacked-sequence {
                      frame #0 {
                        w485 = 0
                        w484 = 2
                        n448 = property on="Radio_Baud(E_U)" class="Bool (严格)"("Disabled"=w484) -> ()  [unwired: 2 in, 2 out]
                        n449 = property on="Baud(E_U)" class="Ring (严格)"("Disabled"=w484) -> ()  [unwired: 2 in, 2 out]
                        n450 = property on="滤波起始ID" class="DigNum (严格)"("Disabled"=w484) -> ()  [unwired: 2 in, 2 out]
                        n451 = property on="滤波结束ID" class="DigNum (严格)"("Disabled"=w484) -> ()  [unwired: 2 in, 2 out]
                        n452 = property on="滤波模式" class="Ring (严格)"("Disabled"=w484) -> ()  [unwired: 2 in, 2 out]
                        n453 = property on="寄存器" class="DigNum (严格)"("Disabled"=w484) -> ()  [unwired: 2 in, 2 out]
                        n454 = property on="验收码" class="DigNum (严格)"("Disabled"=w485) -> ()  [unwired: 2 in, 2 out]
                        n455 = property on="Baud" class="Ring (严格)"("Disabled"=w485) -> ()  [unwired: 2 in, 2 out]
                        n456 = property on="屏蔽码" class="DigNum (严格)"("Disabled"=w485) -> ()  [unwired: 2 in, 2 out]
                        n457 = property on="滤波方式" class="Ring (严格)"("Disabled"=w485) -> ()  [unwired: 2 in, 2 out]
                        n458 = property on="BTR0" class="DigNum (严格)"("Disabled"=w485) -> ()  [unwired: 2 in, 2 out]
                        n459 = property on="BTR1" class="DigNum (严格)"("Disabled"=w485) -> ()  [unwired: 2 in, 2 out]
                        n460 = property on="模式" class="Ring (严格)"("Disabled"=w485) -> ()  [unwired: 2 in, 2 out]
                        n461 = property on="Radio_Baud" class="Bool (严格)"("Disabled"=w485) -> ()  [unwired: 2 in, 2 out]
                      }
                      frame #1 {
                        n462 = local read "Radio_Baud"() -> (w486:bool)
                        n463 = case shown="假" w486 {
                          frame False {
                            w488 = 2
                            n464 = property on="BTR0" class="DigNum (严格)"("Disabled"=w488) -> ()  [unwired: 2 in, 2 out]
                            n465 = property on="BTR1" class="DigNum (严格)"("Disabled"=w488) -> ()  [unwired: 2 in, 2 out]
                            n466 = property on="Baud" class="Ring (严格)"("Disabled"=0) -> ()  [unwired: 2 in, 2 out]
                          }
                          frame True {
                            w490 = 0
                            n467 = property on="BTR0" class="DigNum (严格)"("Disabled"=w490) -> ()  [unwired: 2 in, 2 out]
                            n468 = property on="BTR1" class="DigNum (严格)"("Disabled"=w490) -> ()  [unwired: 2 in, 2 out]
                            n469 = property on="Baud" class="Ring (严格)"("Disabled"=2) -> ()  [unwired: 2 in, 2 out]
                          }
                        }
                      }
                      frame #2 {
                        n470 = local read "Baud"() -> (w491:u32)
                        n471 = case shown="3" w491 {
                          frame 0 {
                            n472 = local write "BTR0"(u8 191 ("BTR0")) -> ()
                            n473 = local write "BTR1"(u8 255 ("BTR1")) -> ()
                          }
                          frame 1 {
                            n474 = local write "BTR0"(u8 49 ("BTR0")) -> ()
                            n475 = local write "BTR1"(u8 28 ("BTR1")) -> ()
                          }
                          frame 2 {
                            n476 = local write "BTR0"(u8 24 ("BTR0")) -> ()
                            n477 = local write "BTR1"(u8 28 ("BTR1")) -> ()
                          }
                          frame 3 {
                            n478 = local write "BTR1"(u8 255 ("BTR1")) -> ()
                            n479 = local write "BTR0"(u8 135 ("BTR0")) -> ()
                          }
                          frame 4 {
                            n480 = local write "BTR1"(u8 28 ("BTR1")) -> ()
                            n481 = local write "BTR0"(u8 9 ("BTR0")) -> ()
                          }
                          frame 5 {
                            n482 = local write "BTR0"(u8 131 ("BTR0")) -> ()
                            n483 = local write "BTR1"(u8 255 ("BTR1")) -> ()
                          }
                          frame 6 {
                            n484 = local write "BTR1"(u8 28 ("BTR1")) -> ()
                            n485 = local write "BTR0"(u8 4 ("BTR0")) -> ()
                          }
                          frame 7 {
                            n486 = local write "BTR0"(u8 3 ("BTR0")) -> ()
                            n487 = local write "BTR1"(u8 28 ("BTR1")) -> ()
                          }
                          frame 8 {
                            n488 = local write "BTR0"(u8 129 ("BTR0")) -> ()
                            n489 = local write "BTR1"(u8 250 ("BTR1")) -> ()
                          }
                          frame 9 {
                            n490 = local write "BTR1"(u8 28 ("BTR1")) -> ()
                            n491 = local write "BTR0"(u8 1 ("BTR0")) -> ()
                          }
                          frame 10 {
                            n492 = local write "BTR0"(u8 128 ("BTR0")) -> ()
                            n493 = local write "BTR1"(u8 250 ("BTR1")) -> ()
                          }
                          frame 11 {
                            n494 = local write "BTR0"(u8 0 ("BTR0")) -> ()
                            n495 = local write "BTR1"(u8 28 ("BTR1")) -> ()
                          }
                          frame 12 {
                            n496 = local write "BTR0"(u8 128 ("BTR0")) -> ()
                            n497 = local write "BTR1"(u8 182 ("BTR1")) -> ()
                          }
                          frame 13 {
                            n498 = local write "BTR1"(u8 22 ("BTR1")) -> ()
                            n499 = local write "BTR0"(u8 0 ("BTR0")) -> ()
                          }
                          frame 14 {
                            n500 = local write "BTR0"(u8 0 ("BTR0")) -> ()
                            n501 = local write "BTR1"(u8 20 ("BTR1")) -> ()
                          }
                          frame 15, Default {
                          }
                        }
                      }
                    }
                  }
                  frame True {
                    w524 = 0
                    w522 = 2
                    n502 = property on="Baud(E_U)" class="Ring (严格)"("Disabled"=w524) -> ()  [unwired: 2 in, 2 out]
                    n503 = property on="滤波起始ID" class="DigNum (严格)"("Disabled"=w524) -> ()  [unwired: 2 in, 2 out]
                    n504 = property on="滤波结束ID" class="DigNum (严格)"("Disabled"=w524) -> ()  [unwired: 2 in, 2 out]
                    n505 = property on="滤波模式" class="Ring (严格)"("Disabled"=w524) -> ()  [unwired: 2 in, 2 out]
                    n506 = property on="Radio_Baud(E_U)" class="Bool (严格)"("Disabled"=w524) -> ()  [unwired: 2 in, 2 out]
                    n507 = local write "Radio_Baud(E_U)"(FALSE) -> ()
                    n508 = local write "BTR1"(u8 0 ("BTR1")) -> ()
                    n509 = local write "BTR0"(u8 0 ("BTR0")) -> ()
                    n510 = property on="寄存器" class="DigNum (严格)"("Disabled"=w522) -> ()  [unwired: 2 in, 2 out]
                    n511 = property on="验收码" class="DigNum (严格)"("Disabled"=w522) -> ()  [unwired: 2 in, 2 out]
                    n512 = property on="滤波方式" class="Ring (严格)"("Disabled"=w522) -> ()  [unwired: 2 in, 2 out]
                    n513 = property on="屏蔽码" class="DigNum (严格)"("Disabled"=w522) -> ()  [unwired: 2 in, 2 out]
                    n514 = property on="BTR0" class="DigNum (严格)"("Disabled"=w522) -> ()  [unwired: 2 in, 2 out]
                    n515 = property on="BTR1" class="DigNum (严格)"("Disabled"=w522) -> ()  [unwired: 2 in, 2 out]
                    n516 = property on="模式" class="Ring (严格)"("Disabled"=w522) -> ()  [unwired: 2 in, 2 out]
                    n517 = property on="Radio_Baud" class="Bool (严格)"("Disabled"=w522) -> ()  [unwired: 2 in, 2 out]
                    n518 = property on="Baud" class="Ring (严格)"("Disabled"=w522) -> ()  [unwired: 2 in, 2 out]
                  }
                }
              }
            }
          }
        }
      }
      event "设备类型": Value Change {
        n519 = event-data() -> ()  [unwired: 7 out]
        n520 = stacked-sequence {
          frame #0 {
            n521 = local read "设备类型"() -> (w529:u32)
            n522 = Quotient & Remainder(x=w529, y=10000) -> (x-y*floor(x/y)=w527:u32)  [unwired: 1 out]
            n523 = local write "设备类型值"(w527) -> ()
          }
          frame #1 {
            w532 = u32 21 items=["PCI5121"=1, "PCI9810"=2, "USBCAN1"=3, "USBCAN2"=4, "PCI9820"=5, "PCI5110"=7, "CANLite(mini)"=8, "ISA9620"=9, "ISA5420"=10, "PC104CAN"=11, "DNP9810"=13, "PCI9840B"=14, "PC104C2"=15, "PCI9820I"=16, "pec9920"=18, "USBCAN_E_U"=20, "USBCAN_2E_U"=21, ""=0] ("DeviceType")
            n524 = local read "设备类型值"() -> (w533:u32)
            n525 = Equal?(x=w532, y=w533) -> (x = y?=w531:bool)
            n526 = case shown="假" w531 {
              tunnel: [T9."Disabled and Grayed Out" ("禁用") T9."Enabled" ("禁用")] -> w530
              frame False {
              }
              frame True {
              }
            }
            n527 = property on="清除定时发送" class="Bool"("DisabledEnum"=w530) -> ()  [unwired: 2 in, 2 out]
            n528 = property on="定时发送" class="Bool"("DisabledEnum"=w530) -> ()  [unwired: 2 in, 2 out]
          }
          frame #2 {
            w542 = u32 22 items=["PCI5121"=1, "PCI9810"=2, "USBCAN1"=3, "USBCAN2"=4, "PCI9820"=5, "PCI5110"=7, "CANLite(mini)"=8, "ISA9620"=9, "ISA5420"=10, "PC104CAN"=11, "DNP9810"=13, "PCI9840B"=14, "PC104C2"=15, "PCI9820I"=16, "pec9920"=18, "PCI5010U"=19, "USBCAN_E_U"=20, "USBCAN_2E_U"=21, "PCI5020U"=22, ""=0] ("DeviceType")
            w543 = u32 19 items=["PCI5121"=1, "PCI9810"=2, "USBCAN1"=3, "USBCAN2"=4, "PCI9820"=5, "PCI5110"=7, "CANLite(mini)"=8, "ISA9620"=9, "ISA5420"=10, "PC104CAN"=11, "DNP9810"=13, "PCI9840B"=14, "PC104C2"=15, "PCI9820I"=16, "pec9920"=18, "PCI5010U"=19, "USBCAN_E_U"=20, "USBCAN_2E_U"=21, "PCI5020U"=22, ""=0] ("DeviceType")
            w546 = u32 21 items=["PCI5121"=1, "PCI9810"=2, "USBCAN1"=3, "USBCAN2"=4, "PCI9820"=5, "PCI5110"=7, "CANLite(mini)"=8, "ISA9620"=9, "ISA5420"=10, "PC104CAN"=11, "DNP9810"=13, "PCI9840B"=14, "PC104C2"=15, "PCI9820I"=16, "pec9920"=18, "USBCAN_E_U"=20, "USBCAN_2E_U"=21, ""=0] ("DeviceType")
            w547 = u32 20 items=["PCI5121"=1, "PCI9810"=2, "USBCAN1"=3, "USBCAN2"=4, "PCI9820"=5, "PCI5110"=7, "CANLite(mini)"=8, "ISA9620"=9, "ISA5420"=10, "PC104CAN"=11, "DNP9810"=13, "PCI9840B"=14, "PC104C2"=15, "PCI9820I"=16, "pec9920"=18, "USBCAN_E_U"=20, "USBCAN_2E_U"=21, ""=0] ("DeviceType")
            n529 = local read "设备类型值"() -> (w541:u32)
            n530 = Equal?(x=w541, y=w547) -> (x = y?=w545:bool)
            n531 = Equal?(x=w541, y=w546) -> (x = y?=w544:bool)
            n532 = Equal?(x=w543, y=w541) -> (x = y?=w540:bool)
            n533 = Equal?(x=w542, y=w541) -> (x = y?=w539:bool)
            n534 = Or(x=w545, y=w544) -> (x .or. y?=w538:bool)
            n535 = Or(x=w540, y=w539) -> (x .or. y?=w537:bool)
            n536 = Or(x=w538, y=w537) -> (x .or. y?=w536:bool)
            n537 = case shown="假" w536 {
              frame False {
                n538 = stacked-sequence {
                  frame #0 {
                    w550 = 0
                    w548 = 2
                    n539 = property on="Baud(E_U)" class="Ring (严格)"("Disabled"=w548) -> ()  [unwired: 2 in, 2 out]
                    n540 = property on="滤波起始ID" class="DigNum (严格)"("Disabled"=w548) -> ()  [unwired: 2 in, 2 out]
                    n541 = property on="滤波结束ID" class="DigNum (严格)"("Disabled"=w548) -> ()  [unwired: 2 in, 2 out]
                    n542 = property on="滤波模式" class="Ring (严格)"("Disabled"=w548) -> ()  [unwired: 2 in, 2 out]
                    n543 = property on="Radio_Baud(E_U)" class="Bool (严格)"("Disabled"=w548) -> ()  [unwired: 2 in, 2 out]
                    n544 = property on="寄存器" class="DigNum (严格)"("Disabled"=w548) -> ()  [unwired: 2 in, 2 out]
                    n545 = property on="BTR0" class="DigNum (严格)"("Disabled"=w548) -> ()  [unwired: 2 in, 2 out]
                    n546 = property on="BTR1" class="DigNum (严格)"("Disabled"=w548) -> ()  [unwired: 2 in, 2 out]
                    n547 = local write "Radio_Baud"(FALSE) -> ()
                    n548 = property on="验收码" class="DigNum (严格)"("Disabled"=w550) -> ()  [unwired: 2 in, 2 out]
                    n549 = property on="屏蔽码" class="DigNum (严格)"("Disabled"=w550) -> ()  [unwired: 2 in, 2 out]
                    n550 = property on="滤波方式" class="Ring (严格)"("Disabled"=w550) -> ()  [unwired: 2 in, 2 out]
                    n551 = property on="BTR0" class="DigNum (严格)"("Disabled"=w550) -> ()  [unwired: 2 in, 2 out]
                    n552 = property on="BTR1" class="DigNum (严格)"("Disabled"=w550) -> ()  [unwired: 2 in, 2 out]
                    n553 = property on="模式" class="Ring (严格)"("Disabled"=w550) -> ()  [unwired: 2 in, 2 out]
                    n554 = property on="Radio_Baud" class="Bool (严格)"("Disabled"=w550) -> ()  [unwired: 2 in, 2 out]
                    n555 = property on="Baud" class="Ring (严格)"("Disabled"=w550) -> ()  [unwired: 2 in, 2 out]
                  }
                  frame #1 {
                    n556 = local read "Baud"() -> (w551:u32)
                    n557 = case shown="0" w551 {
                      frame 0 {
                        n558 = local write "BTR0"(u8 191 ("BTR0")) -> ()
                        n559 = local write "BTR1"(u8 255 ("BTR1")) -> ()
                      }
                      frame 1 {
                        n560 = local write "BTR0"(u8 49 ("BTR0")) -> ()
                        n561 = local write "BTR1"(u8 28 ("BTR1")) -> ()
                      }
                      frame 2 {
                        n562 = local write "BTR0"(u8 24 ("BTR0")) -> ()
                        n563 = local write "BTR1"(u8 28 ("BTR1")) -> ()
                      }
                      frame 3 {
                        n564 = local write "BTR1"(u8 255 ("BTR1")) -> ()
                        n565 = local write "BTR0"(u8 135 ("BTR0")) -> ()
                      }
                      frame 4 {
                        n566 = local write "BTR1"(u8 28 ("BTR1")) -> ()
                        n567 = local write "BTR0"(u8 9 ("BTR0")) -> ()
                      }
                      frame 5 {
                        n568 = local write "BTR0"(u8 131 ("BTR0")) -> ()
                        n569 = local write "BTR1"(u8 255 ("BTR1")) -> ()
                      }
                      frame 6 {
                        n570 = local write "BTR1"(u8 28 ("BTR1")) -> ()
                        n571 = local write "BTR0"(u8 4 ("BTR0")) -> ()
                      }
                      frame 7 {
                        n572 = local write "BTR0"(u8 3 ("BTR0")) -> ()
                        n573 = local write "BTR1"(u8 28 ("BTR1")) -> ()
                      }
                      frame 8 {
                        n574 = local write "BTR0"(u8 129 ("BTR0")) -> ()
                        n575 = local write "BTR1"(u8 250 ("BTR1")) -> ()
                      }
                      frame 9 {
                        n576 = local write "BTR1"(u8 28 ("BTR1")) -> ()
                        n577 = local write "BTR0"(u8 1 ("BTR0")) -> ()
                      }
                      frame 10 {
                        n578 = local write "BTR0"(u8 128 ("BTR0")) -> ()
                        n579 = local write "BTR1"(u8 250 ("BTR1")) -> ()
                      }
                      frame 11 {
                        n580 = local write "BTR0"(u8 0 ("BTR0")) -> ()
                        n581 = local write "BTR1"(u8 28 ("BTR1")) -> ()
                      }
                      frame 12 {
                        n582 = local write "BTR0"(u8 128 ("BTR0")) -> ()
                        n583 = local write "BTR1"(u8 182 ("BTR1")) -> ()
                      }
                      frame 13 {
                        n584 = local write "BTR1"(u8 22 ("BTR1")) -> ()
                        n585 = local write "BTR0"(u8 0 ("BTR0")) -> ()
                      }
                      frame 14 {
                        n586 = local write "BTR0"(u8 0 ("BTR0")) -> ()
                        n587 = local write "BTR1"(u8 20 ("BTR1")) -> ()
                      }
                      frame 15, Default {
                      }
                    }
                  }
                }
              }
              frame True {
                n588 = stacked-sequence {
                  frame #0 {
                    w584 = 0
                    w582 = 2
                    n589 = property on="Baud(E_U)" class="Ring (严格)"("Disabled"=w584) -> ()  [unwired: 2 in, 2 out]
                    n590 = property on="滤波起始ID" class="DigNum (严格)"("Disabled"=w584) -> ()  [unwired: 2 in, 2 out]
                    n591 = property on="滤波结束ID" class="DigNum (严格)"("Disabled"=w584) -> ()  [unwired: 2 in, 2 out]
                    n592 = property on="滤波模式" class="Ring (严格)"("Disabled"=w584) -> ()  [unwired: 2 in, 2 out]
                    n593 = property on="Radio_Baud(E_U)" class="Bool (严格)"("Disabled"=w584) -> ()  [unwired: 2 in, 2 out]
                    n594 = property on="验收码" class="DigNum (严格)"("Disabled"=w582) -> ()  [unwired: 2 in, 2 out]
                    n595 = property on="滤波方式" class="Ring (严格)"("Disabled"=w582) -> ()  [unwired: 2 in, 2 out]
                    n596 = property on="屏蔽码" class="DigNum (严格)"("Disabled"=w582) -> ()  [unwired: 2 in, 2 out]
                    n597 = property on="BTR0" class="DigNum (严格)"("Disabled"=w582) -> ()  [unwired: 2 in, 2 out]
                    n598 = property on="BTR1" class="DigNum (严格)"("Disabled"=w582) -> ()  [unwired: 2 in, 2 out]
                    n599 = property on="模式" class="Ring (严格)"("Disabled"=w582) -> ()  [unwired: 2 in, 2 out]
                    n600 = property on="Radio_Baud" class="Bool (严格)"("Disabled"=w582) -> ()  [unwired: 2 in, 2 out]
                    n601 = property on="Baud" class="Ring (严格)"("Disabled"=w582) -> ()  [unwired: 2 in, 2 out]
                    n602 = property on="寄存器" class="DigNum (严格)"("Disabled"=w582) -> ()  [unwired: 2 in, 2 out]
                    n603 = local write "Radio_Baud(E_U)"(FALSE) -> ()
                    n604 = local write "BTR1"(u8 0 ("BTR1")) -> ()
                    n605 = local write "BTR0"(u8 0 ("BTR0")) -> ()
                  }
                  frame #1 {
                    n606 = local read "Baud(E_U)"() -> (w587:u32)
                    n607 = case shown="60003" w587 {
                      frame 286331153, Default {
                      }
                      frame 393219 {
                        n608 = local write "寄存器"(393219) -> ()
                      }
                      frame 393220 {
                        n609 = local write "寄存器"(393220) -> ()
                      }
                      frame 393223 {
                        n610 = local write "寄存器"(393223) -> ()
                      }
                      frame 1835016 {
                        n611 = local write "寄存器"(1835016) -> ()
                      }
                      frame 1835025 {
                        n612 = local write "寄存器"(1835025) -> ()
                      }
                      frame 1441827 {
                        n613 = local write "寄存器"(1441827) -> ()
                      }
                      frame 1835052 {
                        n614 = local write "寄存器"(1835052) -> ()
                      }
                      frame 1441971 {
                        n615 = local write "寄存器"(1441971) -> ()
                      }
                      frame 1835232 {
                        n616 = local write "寄存器"(1835232) -> ()
                      }
                      frame 1835457 {
                        n617 = local write "寄存器"(1835457) -> ()
                      }
                    }
                  }
                }
              }
            }
          }
        }
      }
      event "StartCAN": Value Change {
        n618 = event-data() -> ()  [unwired: 7 out]
        n619 = local read "设备类型值"() -> (w603:u32)
        n620 = local read "CAN 通道"() -> (w602:u32)
        n621 = local read "索引"() -> (w598:u32)
        n622 = dll-call lib="E:/Project/CANMaster/LabView/ControlCAN_labview/bin/ControlCAN.dll" fn="VCI_StartCAN"("DeviceType"=w603, "DeviceInd"=w598, "CANInd"=w602) -> (w601:u32)  [unwired: 6 in, 2 out]
        n623 = Equal?(x=w601, y=u32 1) -> (x = y?=w599:bool)
        n624 = case shown="真" w599 {
          selector: w599 -> [_ w605]
          frame False {
          }
          frame True {
            w604 = u8 2 ("Disabled")
            n625 = property on="索引" class="Ring (严格)"("Disabled"=w604) -> ()  [unwired: 2 in, 2 out]
            n626 = property on="CAN 通道" class="Ring (严格)"("禁用"=w604) -> ()  [unwired: 2 in, 2 out]
            "CANStartup" <- w605
          }
        }
      }
      event "ResetCAN": Value Change {
        n627 = event-data() -> ()  [unwired: 7 out]
        n628 = local read "索引"() -> (w606:u32)
        n629 = local read "设备类型值"() -> (w611:u32)
        n630 = local read "CAN 通道"() -> (w610:u32)
        n631 = local write "CANStartup"(FALSE) -> ()
        n632 = dll-call lib="E:/Project/CANMaster/LabView/ControlCAN_labview/bin/ControlCAN.dll" fn="VCI_ResetCAN"("DeviceType"=w611, "DeviceInd"=w606, "CANInd"=w610) -> (w609:u32)  [unwired: 6 in, 2 out]
        n633 = Equal?(x=w609, y=u32 1) -> (x = y?=w607:bool)
        n634 = case shown="真" w607 {
          frame False {
          }
          frame True {
            w613 = u8 0 ("Disabled")
            n635 = property on="索引" class="Ring (严格)"("Disabled"=w613) -> ()  [unwired: 2 in, 2 out]
            n636 = property on="CAN 通道" class="Ring (严格)"("禁用"=w613) -> ()  [unwired: 2 in, 2 out]
          }
        }
      }
      event "Clear Buffer": Value Change {
        n637 = event-data() -> ()  [unwired: 2 out]
        n638 = local read "DeviceOpen"() -> (w615:bool)
        n639 = case shown="真" w615 {
          frame False {
          }
          frame True {
            n640 = local read "设备类型值"() -> (w618:u32)
            n641 = local read "CAN 通道"() -> (w617:u32)
            n642 = local read "索引"() -> (w616:u32)
            n643 = dll-call lib="E:/Project/CANMaster/LabView/ControlCAN_labview/bin/ControlCAN.dll" fn="VCI_ClearBuffer"("DeviceType"=w618, "DeviceInd"=w616, "CANInd"=w617) -> ()  [unwired: 6 in, 3 out]
          }
        }
        n644 = property on="Multicolumn Listbox" class="MCListbox (严格)"("项名"=string[][] [] ("t")) -> ()  [unwired: 2 in, 2 out]
      }
      event "GetBoardInfo": Value Change {
        n645 = event-data() -> ()  [unwired: 7 out]
        n646 = local read "设备类型值"() -> (w621:u32)
        n647 = dll-call lib="E:/Project/CANMaster/LabView/ControlCAN_labview/bin/ControlCAN.dll" fn="VCI_ReadBoardInfo"("DeviceType"=u32 0, "DeviceInd"=w621) -> ("VCI_BOARD_INFO"=w619:T2)  [unwired: 5 in, 4 out]
        "VCI_BOARD_INFO" <- w619
        n648 = call "boardinfo.vi"("VCI_BOARD_INFO"=w619) -> ()  [unwired: 1 out]
      }
      event "GetErrorInfo": Value Change {
        n649 = event-data() -> ()  [unwired: 7 out]
        n650 = disable-structure shown="禁用" {
          frame Disabled {
            n651 = local read "设备类型值"() -> (w625:u32)
            n652 = local read "CAN 通道"() -> (w624:u32)
            n653 = local read "索引"() -> (w622:u32)
            n654 = dll-call lib="E:/Project/CANMaster/LabView/ControlCAN_labview/bin/ControlCAN.dll" fn="VCI_ReadErrInfo"("DeviceType"=w625, "DeviceInd"=w622, "CANInd"=w624) -> ("VCI_ERR_INFO"=w623:T3)  [unwired: 6 in, 4 out]
            "VCI_ERR_INFO" <- w623
            n655 = call "errinfo.vi"("VCI_ERR_INFO"=w623) -> ()  [unwired: 1 out]
          }
          frame Enabled {
          }
        }
        n656 = call "ErrFrmRatio.vi"() -> ()  [unwired: 12 in]
      }
      event "总线利用率": Value Change {
        n657 = event-data() -> ()  [unwired: 7 out]
        n658 = global read "globe.vi" "总线利用率视图已打开"() -> (w626:bool)
        n659 = case shown="假" w626 {
          frame False {
            n660 = global write "globe.vi" "总线利用率视图已打开"(TRUE) -> ()
            n661 = Open VI Reference(type specifier VI Refnum (for type only)=refnum<vi> refnum ("类型说明符VI引用句柄（仅用于类型）"), vi path=path "BusRatio.vi" ("VI路径"), options=128 ("选项")) -> (vi reference=w632:refnum<vi>, error out=w631:errorcluster)  [unwired: 3 in]
            n662 = call-by-ref "开始异步调用"(reference=w632, error in=w631) -> (reference out=w630:refnum<vi>, error out=w629:errorcluster)  [unwired: 12 in]
            n663 = Close Reference(reference=w630, error in (no error)=w629) -> (error out=w628:errorcluster)
            n664 = call <vilib>:"Simple Error Handler.vi"("error in (no error)"=w628) -> ()  [unwired: 4 in, 5 out]
          }
          frame True {
          }
        }
      }
      event "GetStatus": Value Change {
        n665 = event-data() -> ()  [unwired: 7 out]
        n666 = local read "设备类型值"() -> (w639:u32)
        n667 = local read "CAN 通道"() -> (w638:u32)
        n668 = local read "索引"() -> (w636:u32)
        n669 = dll-call lib="E:/Project/CANMaster/LabView/ControlCAN_labview/bin/ControlCAN.dll" fn="VCI_ReadCANStatus"("DeviceType"=w639, "DeviceInd"=w636, "CANInd"=w638) -> ("VCI_CAN_STATUS"=w637:T4)  [unwired: 6 in, 4 out]
        "VCI_CAN_STATUS" <- w637
        n670 = call "status.vi"("VCI_CAN_STATUS"=w637) -> ()  [unwired: 1 out]
      }
      event User Event {
        n671 = event-data() -> ("Tx_Or_Rx"=w642:bool, "VCI_CAN_OBJ_N"=w641:T1, "Num"=w640:u32)  [unwired: 2 out]
        n672 = for {
          N: w640 -> [_]
          tunnel: w641 -> [w644] mode=indexing
          tunnel: w642 -> [w660]
          w689 = 2
          w710 = 8
          n673 = Unbundle(w644) -> ("ID"=w712:u32, "TimeStamp"=w709:u32, "TimeFlag"=w690:u8, "SendType"=w707:u8, "RemoteFlag"=w708:u8, "ExternFlag"=w706:u8, "DataLen"=w678:u8, w699:u8, w698:u8, w697:u8, w696:u8, w695:u8, w694:u8, w692:u8, w693:u8)  [unwired: 3 out]
          n674 = local read "TRCount"() -> (w663:u32)
          n675 = Build Array(w699, w698, w697, w696, w695, w694, w692, w693) -> (w679:u8[])
          n676 = Select(t="T", s=w660, f="R") -> (s? t:f=w659:string)
          n677 = Increment(x=w663) -> (x+1=→"TRCount":u32)
          n678 = Number To Hexadecimal String(1:w710, 2:w712) -> (0:w711:string)
          n679 = Number To Decimal String(number=w709, width (-)=w710) -> (decimal integer string=w705:string)
          n680 = Number To Hexadecimal String(1:w689, 2:w690) -> (0:w691:string)
          n681 = Number To Hexadecimal String(1:w689, 2:w707) -> (0:w704:string)
          n682 = Number To Hexadecimal String(1:w689, 2:w708) -> (0:w703:string)
          n683 = Number To Hexadecimal String(1:w689, 2:w706) -> (0:w702:string)
          n684 = Number To Decimal String(number=w678, width (-)=1) -> (decimal integer string=w700:string)
          n685 = Number To Decimal String(number=w663, width (-)=i16 8) -> (decimal integer string=w686:string)
          n686 = for {
            N: w678 -> [_]
            shift-right: [w715] -> w681
            shift-left: "" -> [w713]
            tunnel: w679 -> [w714] mode=indexing
            n687 = Number To Hexadecimal String(1:i16 2 ("width (-)"), 2:w714) -> (0:w717:string)
            n688 = Concatenate Strings(w713, w717, " " ("string")) -> (w715:string)
          }
          n689 = Build Array(w686, w659, w711, w705, w691, w704, w703, w702, w700, w681) -> (w688:string[])
          n690 = property on="Multicolumn Listbox" class="MCListbox (严格)"() -> ("项名"=w683:string[][])  [unwired: 2 in, 2 out]
          n691 = local read "Num Rows"() -> (w664:u32)
          n692 = Array Size(array=w683) -> (size(s)=w682:i32[])
          n693 = Index Array(array=w682, index=0) -> (element=w667:i32)
          n694 = Greater Or Equal?(x=w667, y=1000) -> (x >= y?=w677:bool)
          n695 = Insert Into Array(array=w683, index (row)=w667, new element=w688) -> (w675:string[][])  [unwired: 1 in]
          n696 = Decrement(x=w664) -> (x-1=w665:u32)
          n697 = Select(t=string[][] [], s=w677, f=w675) -> (s? t:f=w676:string[][])
          n698 = Greater Or Equal?(x=w667, y=w665) -> (x >= y?=w669:bool)
          n699 = property on="Multicolumn Listbox" class="MCListbox (严格)"("项名"=w676) -> ("行数"=→"Num Rows":u32)  [unwired: 2 in, 2 out]
          n700 = Select(t=w667, s=w669, f=u32 0) -> (s? t:f=w666:u32)
          n701 = Subtract(x=w666, y=w665) -> (x-y=w670:u32)
          n702 = Bundle(w670, u32 0) -> ()  [unwired: 2 out]
          n703 = Unbundle(w644) -> ("RemoteFlag"=w654:u8, "ExternFlag"=w658:u8, "DataLen"=w650:u8)  [unwired: 15 out]
          n704 = Not Equal To 0?(x=w654) -> (x != 0?=w652:bool)
          n705 = Not Equal To 0?(x=w658) -> (x != 0?=w657:bool)
          n706 = Multiply(x=w650, y=8.0) -> (x*y=w649:dbl)
          n707 = Select(t=0, s=w652, f=w649) -> (s? t:f=w648:dbl)
          n708 = global read "globe.vi" "总线比特数"() -> (w645:u64)
          n709 = Select(t=65, s=w657, f=47) -> (s? t:f=w647:i32)
          n710 = Add(x=w648, y=w647) -> (x+y=w646:dbl)
          n711 = Add(x=w646, y=w645) -> (x+y=w643:dbl)
          n712 = global write "globe.vi" "总线比特数"(w643) -> ()
        }
      }
      event "SEND_NCAN": Value Change {
        n713 = event-data() -> ()  [unwired: 7 out]
        n714 = case shown="真" "SEND_NCAN" {
          frame False {
          }
          frame True {
            n715 = stacked-sequence {
              frame #0 {
                n716 = local read "VCI_CAN_OBJ_T"() -> (w721:T6)
                n717 = Build Array(w721, w721, w721, w721, w721, w721, w721, w721, w721, w721, w721, w721, w721) -> (w720:T1)
                n718 = local write "VCI_CAN_OBJ_T_N"(w720) -> ()
              }
              frame #1 {
                n719 = local read "VCI_CAN_OBJ_T_N"() -> (w726:T1)
                n720 = local read "索引"() -> (w722:u32)
                n721 = local read "设备类型值"() -> (w727:u32)
                n722 = local read "CAN 通道"() -> (w728:u32)
                n723 = dll-call lib="E:/Project/CANMaster/LabView/ControlCAN_labview/bin/ControlCAN.dll" fn="VCI_Transmit"("DeviceType"=w727, "DeviceInd"=w722, "CANInd"=w728, "pSend"=w726, "Len"=u32 13) -> ("返回类型"=w724:u32)  [unwired: 8 in, 2 out]
                n724 = Equal?(x=w724, y=u32 13) -> (x = y?=w723:bool)
                n725 = case shown="真" w723 {
                  frame False {
                    n726 = call "显示对话框信息2"() -> ()  [unwired: 3 in, 9 out]
                  }
                  frame True {
                    n727 = call "显示对话框信息"() -> ()  [unwired: 3 in, 9 out]
                  }
                }
              }
            }
          }
        }
      }
      event "Baud(E_U)": Value Change {
        n728 = event-data() -> ()  [unwired: 7 out]
        n729 = local read "Baud(E_U)"() -> (w730:u32)
        n730 = case shown="1C00E0" w730 {
          frame 286331153, Default {
          }
          frame 393219 {
            n731 = local write "寄存器"(393219) -> ()
          }
          frame 393220 {
            n732 = local write "寄存器"(393220) -> ()
          }
          frame 393223 {
            n733 = local write "寄存器"(393223) -> ()
          }
          frame 1835016 {
            n734 = local write "寄存器"(1835016) -> ()
          }
          frame 1835025 {
            n735 = local write "寄存器"(1835025) -> ()
          }
          frame 1441827 {
            n736 = local write "寄存器"(1441827) -> ()
          }
          frame 1835052 {
            n737 = local write "寄存器"(1835052) -> ()
          }
          frame 1441971 {
            n738 = local write "寄存器"(1441971) -> ()
          }
          frame 1835232 {
            n739 = local write "寄存器"(1835232) -> ()
          }
          frame 1835457 {
            n740 = local write "寄存器"(1835457) -> ()
          }
        }
      }
      event "Radio_Baud(E_U)": Value Change {
        n741 = event-data() -> ()  [unwired: 7 out]
        n742 = local read "Radio_Baud(E_U)"() -> (w741:bool)
        n743 = case shown="真" w741 {
          frame False {
            n744 = property on="Baud(E_U)" class="Ring (严格)"("Disabled"=0) -> ()  [unwired: 2 in, 2 out]
            n745 = property on="寄存器" class="DigNum (严格)"("Disabled"=2) -> ()  [unwired: 2 in, 2 out]
          }
          frame True {
            n746 = property on="Baud(E_U)" class="Ring (严格)"("Disabled"=2) -> ()  [unwired: 2 in, 2 out]
            n747 = property on="寄存器" class="DigNum (严格)"("Disabled"=0) -> ()  [unwired: 2 in, 2 out]
          }
        }
      }
    }
  }
  n748 = property on="OpenDevice" class="Bool"("布尔文本.文本"="打开设备" ("Boolean Text.Text")) -> ()  [unwired: 2 in, 2 out]
  n749 = property on="CAN 通道" class="Ring (严格)"("禁用"=w2) -> ()  [unwired: 2 in, 2 out]
  n750 = property on="设备类型值" class="Ring (严格)"("禁用"=w2) -> ()  [unwired: 2 in, 2 out]
  n751 = property on="索引" class="Ring (严格)"("Disabled"=w2) -> ()  [unwired: 2 in, 2 out]
  n752 = local write "CANStartup"(w4) -> ()
  n753 = local write "DeviceOpen"(w4) -> ()
  n754 = local write "CANET IP"("192.168.21.78" ("CANET IP")) -> ()
  n755 = global write "globe.vi" "总线利用率视图已打开"(FALSE) -> ()
  n756 = local write "CANET 端口"(u32 4002 ("CANET 端口")) -> ()
  n757 = while {
    stop <- w746 stop-if-true
    n758 = local read "CANStartup"() -> (w747:bool)
    n759 = case shown="真" w747 {
      frame False {
        n760 = Wait (ms)(milliseconds to wait=u32 50 ("等待时间（毫秒）")) -> ()  [unwired: 1 out]
      }
      frame True {
        n761 = local read "设备类型值"() -> (w754:u32)
        n762 = local read "CAN 通道"() -> (w753:u32)
        n763 = local read "索引"() -> (w752:u32)
        n764 = dll-call lib="E:/Project/CANMaster/LabView/ControlCAN_labview/bin/ControlCAN.dll" fn="VCI_ReadErrInfo"("DeviceType"=w754, "DeviceInd"=w753, "CANInd"=w752) -> ("VCI_ERR_INFO"=w751:T3)  [unwired: 6 in, 4 out]
        n765 = local write "VCI_ERR_INFO"(w751) -> ()
        n766 = Unbundle(w751) -> ("ErrCode"=w749:u32)  [unwired: 4 out]
        n767 = Greater Than 0?(x=w749) -> (x > 0?=w750:bool)
        n768 = case shown="真" w750 {
          tunnel: w749 -> [_ w756]
          frame False {
            n769 = Wait (ms)(milliseconds to wait=u32 50 ("等待时间（毫秒）")) -> ()  [unwired: 1 out]
          }
          frame True {
            # "总线错误"
            n770 = Less?(x=w756, y=u32 256) -> (x < y?=w757:bool)
            n771 = case shown="真" w757 {
              frame False {
              }
              frame True {
                n772 = global read "globe.vi" "总线错误帧数"() -> (w760:u32)
                n773 = Add(x=1.0 ("t"), y=w760) -> (x+y=w761:dbl)
                n774 = global write "globe.vi" "总线错误帧数"(w761) -> ()
              }
            }
          }
        }
      }
    }
    n775 = local read "stop 2"() -> (w746:bool)
  }
  n776 = global write "globe.vi" "发送帧数"(w5) -> ()
  n777 = global write "globe.vi" "接收帧数"(w5) -> ()
  n778 = global write "globe.vi" "总线错误帧数"(w5) -> ()
  n779 = local write "本机端口"(u32 4003 ("本机端口")) -> ()
  n780 = while {
    tunnel: w6 -> [w765]
    tunnel: w23 -> [w764]
    tunnel: [w767] -> w25
    tunnel: [w766] -> w24
    stop <- w762 stop-if-true
    n781 = case shown="真" "Transmit" {
      tunnel: [w769 w779] -> w767
      tunnel: [w770 w778] -> w766
      tunnel: w765 -> [w770 w777]
      tunnel: w764 -> [w769 w776]
      frame False {
        n782 = Wait Until Next ms Multiple(millisecond multiple=u32 10) -> ()  [unwired: 1 out]
      }
      frame True {
        n783 = local read "一次发送帧数"() -> (w775:u32)
        n784 = local read "设备类型值"() -> (w783:u32)
        n785 = local read "CAN 通道"() -> (w782:u32)
        n786 = local read "索引"() -> (w771:u32)
        n787 = for {
          N: w775 -> [_]
          tunnel: [w784] -> w773 mode=indexing
          tunnel: [w784] -> w772
          n788 = local read "VCI_CAN_OBJ_T"() -> (w784:T6)
        }
        n789 = dll-call lib="E:/Project/CANMaster/LabView/ControlCAN_labview/bin/ControlCAN.dll" fn="VCI_Transmit"("DeviceType"=w783, "DeviceInd"=w771, "CANInd"=w782, "pSend"=w773, "Len"=w775) -> ("return type"=w774:u32)  [unwired: 7 in, 3 out]
        n790 = Greater Or Equal?(x=w774, y=u32 1) -> (x >= y?=w780:bool)
        n791 = local write "VCI_CAN_OBJ_TN"(w773) -> ()
        n792 = case shown="真" w780 {
          tunnel: w777 -> [w786 w797]
          tunnel: w776 -> [w785 w796]
          tunnel: [w785 w795] -> w779
          tunnel: [w786 w794] -> w778
          tunnel: w774 -> [_ w789]
          tunnel: w773 -> [_ w791]
          tunnel: w772 -> [_ w790]
          frame False {
            n793 = call "Display Message to User"() -> ()  [unwired: 3 in, 9 out]
          }
          frame True {
            n794 = Bundle(TRUE, "VCI_CAN_OBJ_T"=w790, w791, "return type"=w789) -> (w792:T14)  [unwired: 1 out]
            n795 = Generate User Event(user event=w797, event data cluster=w792, error in=w796) -> (user event out=w794:refnum<user-event>, error out=w795:errorcluster)  [unwired: 1 in]
            n796 = global read "globe.vi" "发送帧数"() -> (w788:u32)
            n797 = Add(x=w788, y=w789) -> (x+y=w787:u32)
            n798 = global write "globe.vi" "发送帧数"(w787) -> ()
          }
        }
      }
    }
    n799 = local read "stop 2"() -> (w762:bool)
  }
  n800 = local write "CANStartup"(FALSE) -> ()
  n801 = local write "TRCount"(u32 0 ("TRCount")) -> ()
  n802 = local write "stop 2"(FALSE ("stop 2")) -> ()
  n803 = Unregister For Events "取消注册事件"(event registration refnum=w26, error in=w25) -> (error out=w29:errorcluster)
  n804 = property on="Multicolumn Listbox" class="MCListbox (严格)"("项名"=string[][] [] ("Item Names")) -> ()  [unwired: 2 in, 2 out]
  n805 = Destroy User Event "销毁用户事件"(user event=w24, error in=w29) -> ()  [unwired: 1 out]
  "type" <- u8[] [1, 0, 0, 0] ("type")
